vi "DG535.ProcCases.vi"(0 "i ref in":refnum<vi>, 1 "selector":string, 2 "Data":T1, 3 "call cluster":T2={"Object"="", "Selector"="", "CallType"=enum."synchronous", "Async Object"="", "Async Selector"="", "Data Descriptor"="", "Data"=[], "Error #"=0, "Expire"=0}, 5 "error in (no error)":errorcluster) -> (14 "i ref out":refnum<vi>, 17 "answer cluster":T2={"Object"="", "Selector"="", "CallType"=enum."synchronous", "Async Object"="", "Async Selector"="", "Data Descriptor"="", "Data"=[], "Error #"=0, "Expire"=0}, 19 "error out":errorcluster)   [LabVIEW 2014, in "DG535.lvlib"]
doc: "This method is called by a process from within the default case in the event loop. The methods of a class that are linked to events will be called from THIS method. Add your code here."
uses:
  DG535.lvlib
  CSCore/BaseProcess/BaseProcess.lvlib
  CSCore/CSSystem/CoreLib/CoreLib.lvlib
  CSCore/CSSystem/CoreLib/CoreLib.string 2 byte array.vi
  CSCore/CSSystem/CoreLib/CoreLib.double 2 byte array.vi
  CSCore/CSSystem/CoreLib/CoreLib.int 2 byte array.vi
  CSCore/CSSystem/CoreLib/CoreLib.byte array 2 int.vi
  CSCore/CSSystem/CoreLib/CoreLib.byte array 2 double.vi
  CSCore/CSSystem/CoreLib/CoreLib.byte array 2 short.vi
  CSCore/CSSystem/CoreLib/CoreLib.byte array 2 string.vi
  CSCore/CSSystem/CoreLib/CoreLib.short 2 byte array.vi
  CSCore/BaseProcess/BaseProcess.descriptor string definition.ctl
  CSCore/CSSystem/CoreDefs/CoreDefs.call_type.ctl
  CSCore/CSSystem/CoreDefs/CoreDefs.rawDataType.ctl
panel:
  in  "error IO":errorcluster
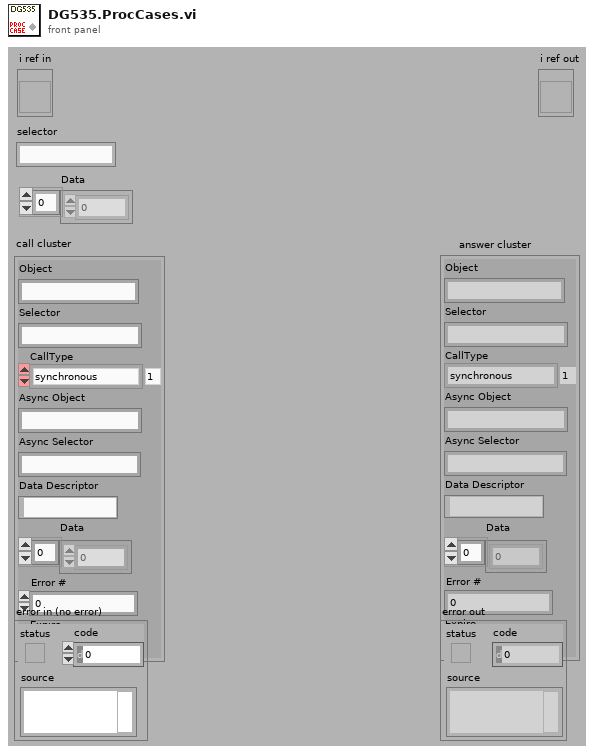
[diagram p1: front panel]
types:
  T1 = typedef "CoreDefs.rawDataType.ctl" = i8[]
  T2 = typedef "CoreDefs.call_type.ctl" = cluster{"Object":string, "Selector":string, "CallType":enum16{"simple", "synchronous", "asynchronous"}, "Async Object":string, "Async Selector":string, "Data Descriptor":T3, "Data":T1, "Error #":i32, "Expire":u32}
  T3 = typedef "BaseProcess.lvlib/BaseProcess.descriptor string definition.ctl" = string
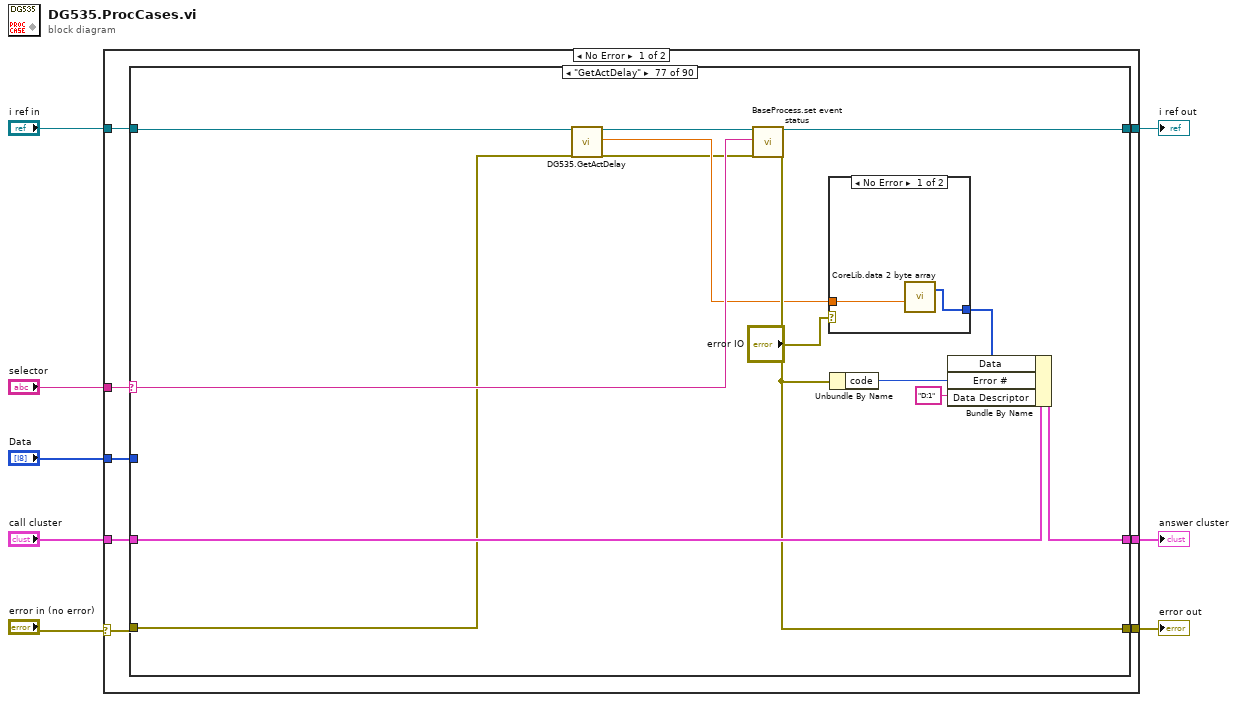
[diagram p0: block diagram]
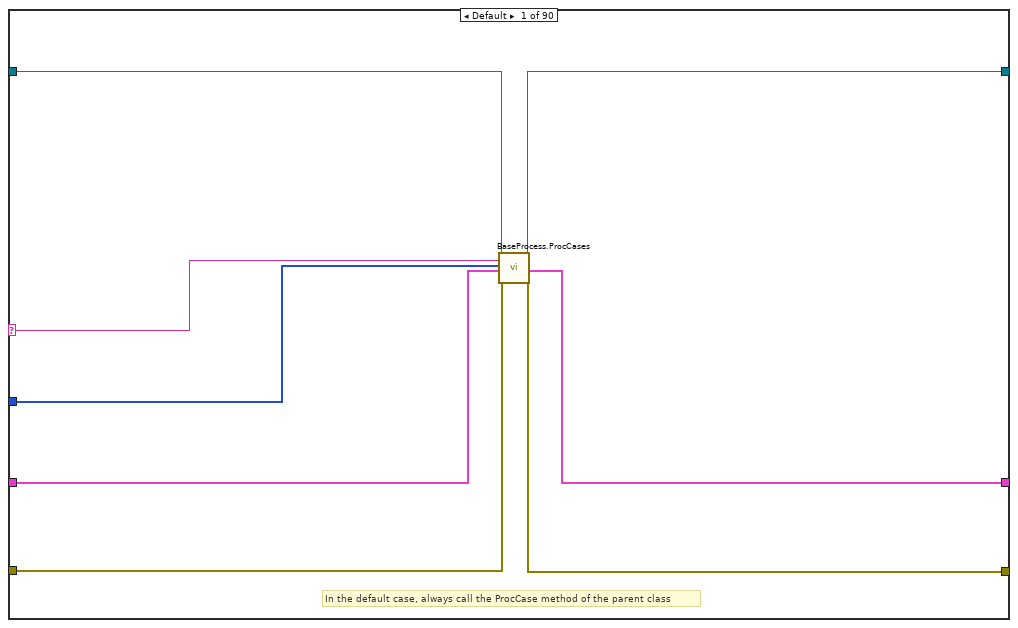
[diagram p2: hidden frame]
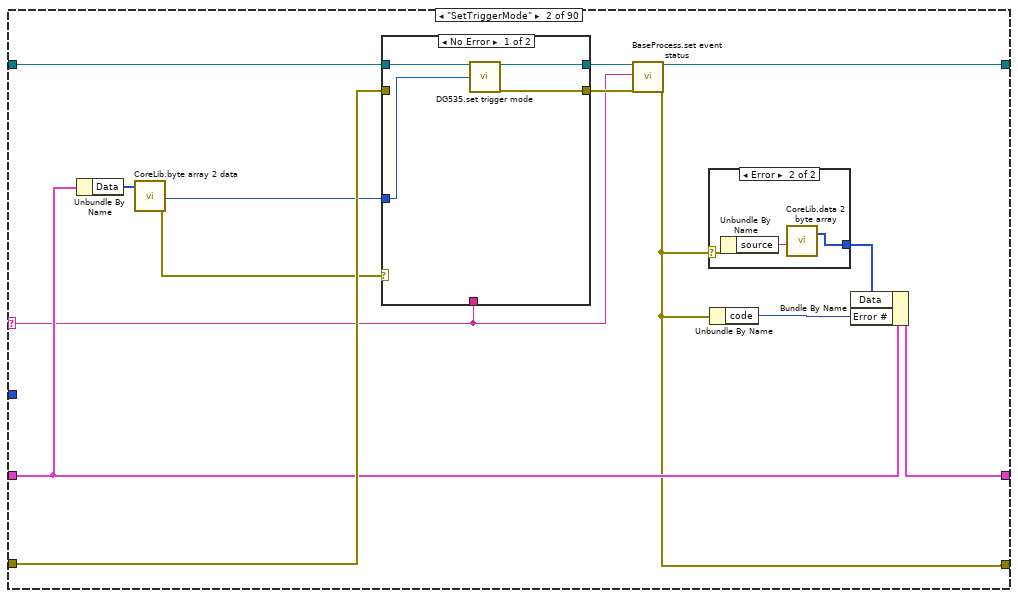
[diagram p3: hidden frame]
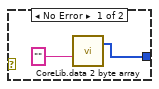
[diagram p4: hidden frame]
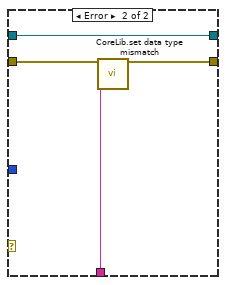
[diagram p5: hidden frame]
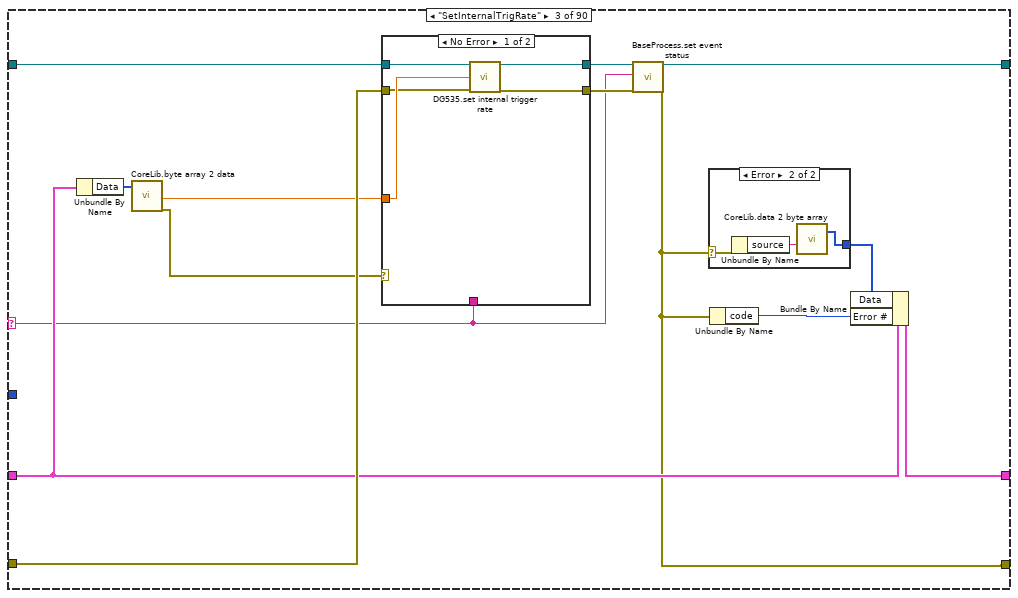
[diagram p6: hidden frame]
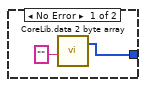
[diagram p7: hidden frame]
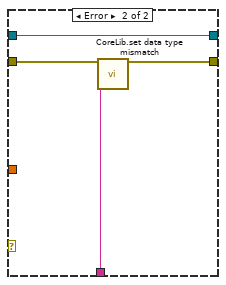
[diagram p8: hidden frame]
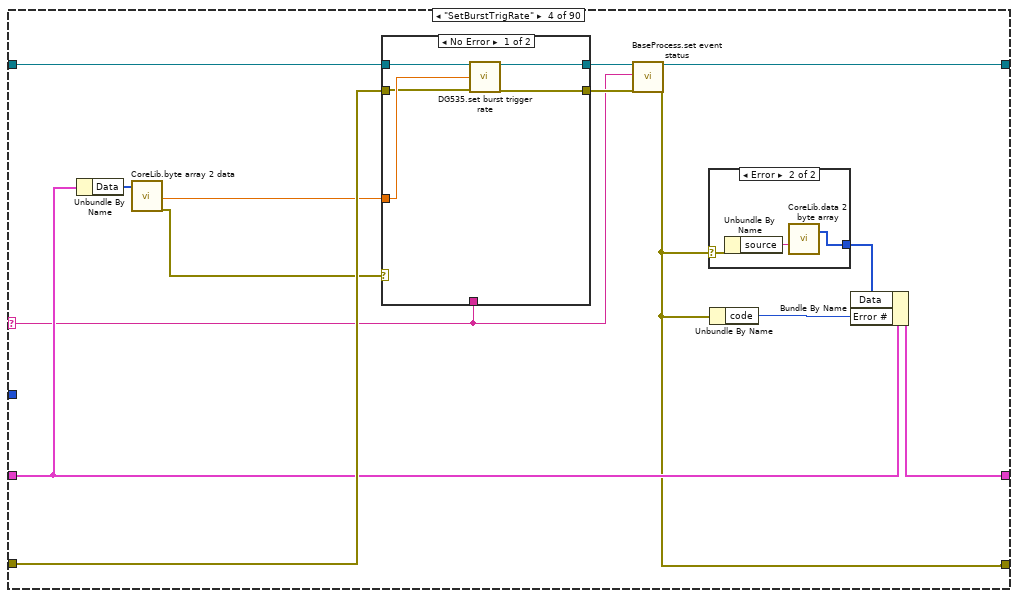
[diagram p9: hidden frame]
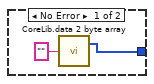
[diagram p10: hidden frame]
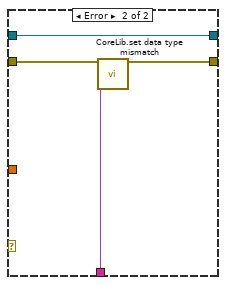
[diagram p11: hidden frame]
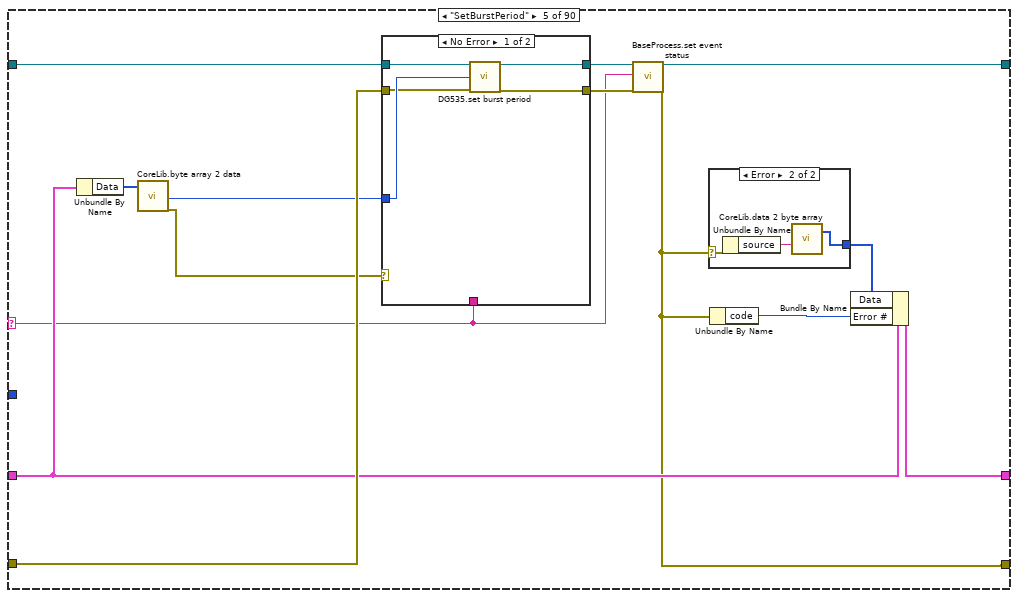
[diagram p12: hidden frame]
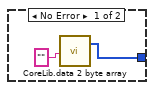
[diagram p13: hidden frame]
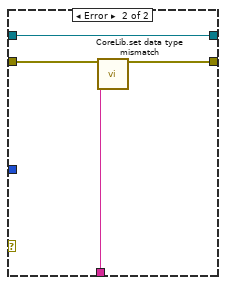
[diagram p14: hidden frame]
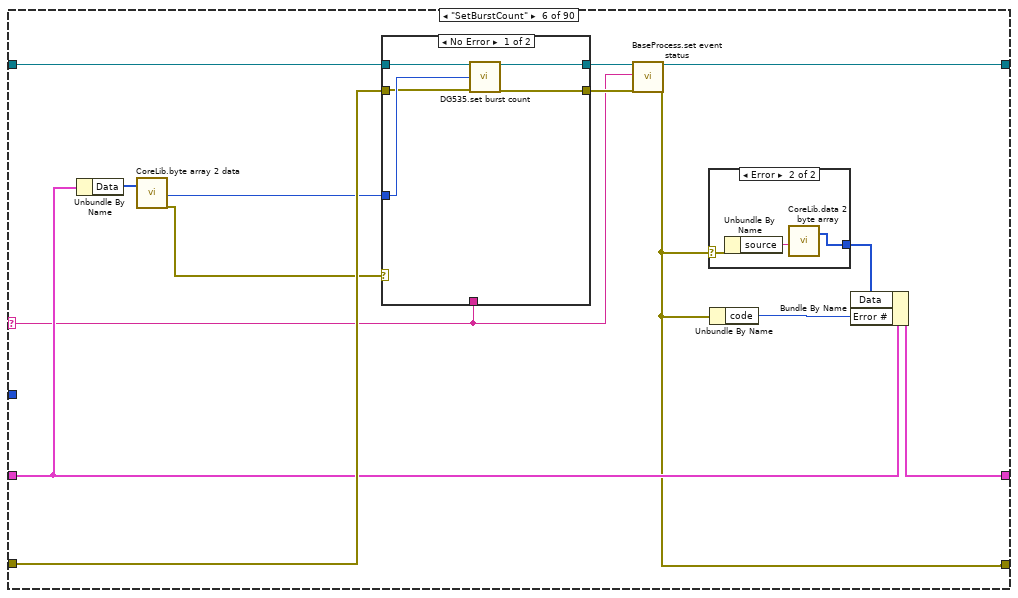
[diagram p15: hidden frame]
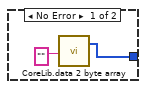
[diagram p16: hidden frame]
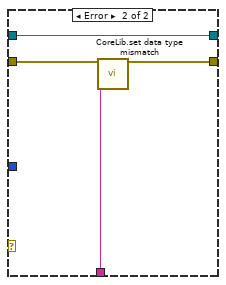
[diagram p17: hidden frame]
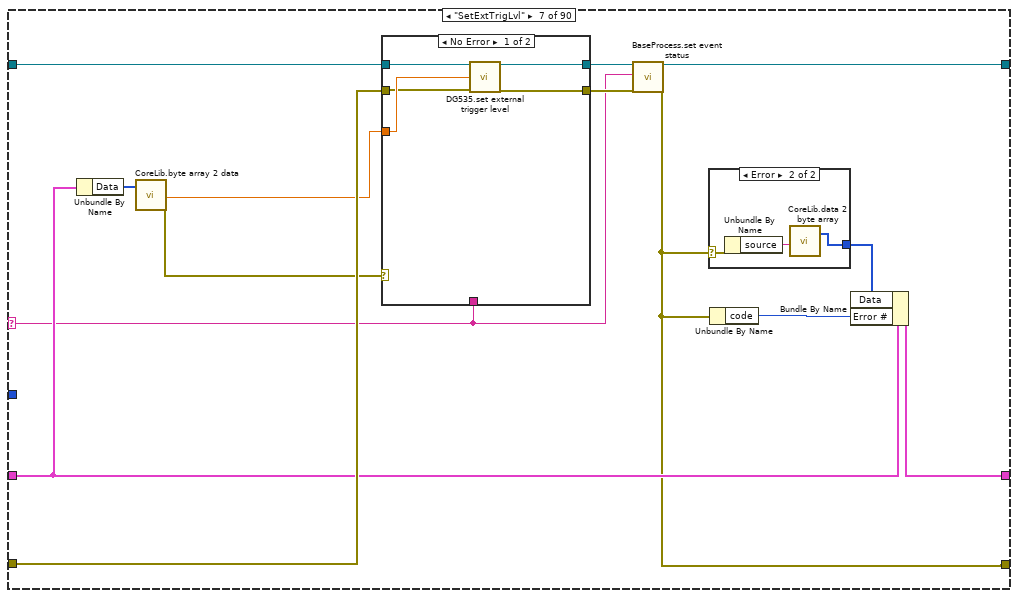
[diagram p18: hidden frame]
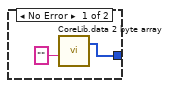
[diagram p19: hidden frame]
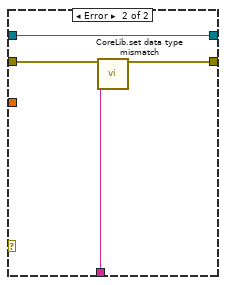
[diagram p20: hidden frame]
diagram:
  n1 = case shown="No Error" "error in (no error)" {
    selector: "error in (no error)" -> [w9 w2268]
    tunnel: "selector" -> [w16 _]
    tunnel: [w15 w2267] -> w7
    tunnel: "call cluster" -> [w14 w2267]
    tunnel: "i ref in" -> [w13 w2269]
    tunnel: [w12 w2269] -> w4
    tunnel: [w11 w2268] -> w3
    tunnel: "Data" -> [w10 _]
    frame No Error {
      n2 = case shown="\"GetActDelay\"" w16 {
        selector: w16 -> [w18 w30 w57 w85 w113 w141 w169 w201 w233 w261 w289 w317 w345 w373 w401 w429 w461 w493 w521 w549 w577 w605 w633 w661 w689 w717 w745 w773 w801 w829 w857 w885 w917 w949 w981 w1013 w1045 w1077 w1109 w1133 w1168 w1200 w1232 w1264 w1296 w1315 w1334 w1353 w1372 w1391 w1410 w1429 w1448 w1467 w1485 w1503 w1521 w1539 w1557 w1575 w1593 w1611 w1629 w1647 w1665 w1683 w1701 w1719 w1737 w1755 w1773 w1791 w1809 w1827 w1863 w1928 w1967 w1985 w2006 w2027 w2047 w2077 w2128 w2147 w2166 w2184 w2202 w2221 w2239 w2257]
        tunnel: w10 -> [w19 _ _ _ _ _ _ _ _ _ _ _ _ _ _ _ _ _ _ _ _ _ _ _ _ _ _ _ _ _ _ _ _ _ _ _ _ _ _ _ _ _ _ _ _ _ _ _ _ _ _ _ _ _ _ _ _ _ _ _ _ _ _ _ _ _ _ _ _ _ _ _ _ _ _ _ _ _ _ _ _ _ _ _ _ _ _ _ _ _]
        tunnel: w13 -> [w17 w38 w65 w93 w121 w149 w177 w209 w241 w269 w297 w325 w353 w381 w409 w437 w469 w501 w529 w557 w585 w613 w641 w669 w697 w725 w753 w781 w809 w837 w865 w893 w925 w957 w989 w1021 w1053 w1085 w1117 w1144 w1176 w1208 w1240 w1272 w1293 w1312 w1331 w1350 w1369 w1388 w1407 w1426 w1445 w1464 w1482 w1500 w1518 w1536 w1554 w1572 w1590 w1608 w1626 w1644 w1662 w1680 w1698 w1716 w1734 w1752 w1770 w1788 w1806 w1824 w1871 w1936 w1961 w1983 w2004 w2025 w2045 w2085 w2125 w2144 w2163 w2181 w2199 w2218 w2236 w2254]
        tunnel: [w24 w29 w56 w84 w112 w140 w168 w200 w232 w260 w288 w316 w344 w372 w400 w428 w460 w492 w520 w548 w576 w604 w632 w660 w688 w716 w744 w772 w800 w828 w856 w884 w916 w948 w980 w1012 w1044 w1076 w1108 w1138 w1167 w1199 w1231 w1263 w1295 w1314 w1333 w1352 w1371 w1390 w1409 w1428 w1447 w1466 w1484 w1502 w1520 w1538 w1556 w1574 w1592 w1610 w1628 w1646 w1664 w1682 w1700 w1718 w1736 w1754 w1772 w1790 w1808 w1826 w1862 w1927 w1963 w1984 w2005 w2026 w2046 w2076 w2127 w2146 w2165 w2183 w2201 w2220 w2238 w2256] -> w12
        tunnel: w14 -> [w20 w35 w62 w90 w118 w146 w174 w206 w238 w266 w294 w322 w350 w378 w406 w434 w466 w498 w526 w554 w582 w610 w638 w666 w694 w722 w750 w778 w806 w834 w862 w890 w922 w954 w986 w1018 w1050 w1082 w1114 w1141 w1173 w1205 w1237 w1269 w1299 w1318 w1337 w1356 w1375 w1394 w1413 w1432 w1451 w1470 w1488 w1506 w1524 w1542 w1560 w1578 w1596 w1614 w1632 w1650 w1668 w1686 w1704 w1722 w1740 w1758 w1776 w1794 w1812 w1830 w1868 w1933 w1966 w1988 w2009 w2030 w2050 w2082 w2132 w2151 w2170 w2188 w2206 w2224 w2242 w2260]
        tunnel: [w21 w34 w61 w89 w117 w145 w173 w205 w237 w265 w293 w321 w349 w377 w405 w433 w465 w497 w525 w553 w581 w609 w637 w665 w693 w721 w749 w777 w805 w833 w861 w889 w921 w953 w985 w1017 w1049 w1081 w1113 w1135 w1172 w1204 w1236 w1268 w1298 w1317 w1336 w1355 w1374 w1393 w1412 w1431 w1450 w1469 w1487 w1505 w1523 w1541 w1559 w1577 w1595 w1613 w1631 w1649 w1667 w1685 w1703 w1721 w1739 w1757 w1775 w1793 w1811 w1829 w1867 w1932 w1965 w1987 w2008 w2029 w2049 w2081 w2131 w2150 w2169 w2187 w2205 w2223 w2241 w2259] -> w15
        tunnel: w9 -> [w23 w37 w64 w92 w120 w148 w176 w208 w240 w268 w296 w324 w352 w380 w408 w436 w468 w500 w528 w556 w584 w612 w640 w668 w696 w724 w752 w780 w808 w836 w864 w892 w924 w956 w988 w1020 w1052 w1084 w1116 w1143 w1175 w1207 w1239 w1271 w1294 w1313 w1332 w1351 w1370 w1389 w1408 w1427 w1446 w1465 w1483 w1501 w1519 w1537 w1555 w1573 w1591 w1609 w1627 w1645 w1663 w1681 w1699 w1717 w1735 w1753 w1771 w1789 w1807 w1825 w1870 w1935 w1962 w1982 w2003 w2024 w2044 w2084 w2126 w2145 w2164 w2182 w2200 w2219 w2237 w2255]
        tunnel: [w22 w31 w58 w86 w114 w142 w170 w202 w234 w262 w290 w318 w346 w374 w402 w430 w462 w494 w522 w550 w578 w606 w634 w662 w690 w718 w746 w774 w802 w830 w858 w886 w918 w950 w982 w1014 w1046 w1078 w1110 w1136 w1169 w1201 w1233 w1265 w1297 w1316 w1335 w1354 w1373 w1392 w1411 w1430 w1449 w1468 w1486 w1504 w1522 w1540 w1558 w1576 w1594 w1612 w1630 w1648 w1666 w1684 w1702 w1720 w1738 w1756 w1774 w1792 w1810 w1828 w1864 w1929 w1964 w1986 w2007 w2028 w2048 w2078 w2129 w2148 w2167 w2185 w2203 w2222 w2240 w2258] -> w11
        frame Default {
          # "In the default case, always call the ProcCase method of the parent class"
          n3 = call "BaseProcess.ProcCases.vi"("i ref in"=w17, "selector"=w18, "Data"=w19, "call cluster"=w20, "error in (no error)"=w23) -> ("i ref out"=w24:refnum<vi>, "answer cluster"=w21:T2, "error out"=w22:errorcluster)  [unwired: 12 in]
        }
        frame "SetTriggerMode" {
          n4 = Unbundle By Name(w35) -> ("Data"=w28:T1)
          n5 = call-poly "CoreLib.byte array 2 data.vi"("byteArray"=w28) -> ("i32"=w27:i32, "error out"=w26:errorcluster)  [unwired: 16 in, 1 out]
          n6 = case shown="No Error" w26 {
            tunnel: [w45 w51] -> w33
            tunnel: w38 -> [w46 w51]
            tunnel: w37 -> [_ w50]
            tunnel: [w44 w49] -> w32
            tunnel: w30 -> [_ w48]
            tunnel: w27 -> [w47 _]
            frame No Error {
              n7 = call "DG535.set trigger mode.vi"("i ref in"=w46, "Trigger Mode"=w47) -> ("i ref out"=w45:refnum<vi>, "error out"=w44:errorcluster)  [unwired: 12 in]
            }
            frame Error {
              n8 = call "CoreLib.set data type mismatch.vi"("error in (no error)"=w50, "error source"=w48) -> ("error out"=w49:errorcluster)  [unwired: 17 in]
            }
          }
          n9 = call "BaseProcess.set event status.vi"("i ref in"=w33, "EventStatus"=w30, "error in (no error)"=w32) -> ("i ref out"=w29:refnum<vi>, "error out"=w31:errorcluster)  [unwired: 14 in, 1 out]
          n10 = case shown="Error" w31 {
            selector: w31 -> [_ w43]
            tunnel: [w39 w41] -> w25
            frame No Error {
              n11 = call-poly "CoreLib.data 2 byte array.vi"("string"="" ("source")) -> ("byteArray out"=w39:T1)  [unwired: 18 in]
            }
            frame Error {
              n12 = Unbundle By Name(w43) -> ("source"=w42:string)
              n13 = call-poly "CoreLib.data 2 byte array.vi"("string"=w42) -> ("byteArray out"=w41:T1)  [unwired: 18 in]
            }
          }
          n14 = Unbundle By Name(w31) -> ("code"=w36:i32)
          n15 = Bundle By Name(cluster=w35, "Data"=w25, "Error #"=w36) -> (w34:T2)
        }
        frame "SetInternalTrigRate" {
          n16 = Unbundle By Name(w62) -> ("Data"=w55:T1)
          n17 = call-poly "CoreLib.byte array 2 data.vi"("byteArray"=w55) -> ("d64"=w54:dbl, "error out"=w53:errorcluster)  [unwired: 16 in, 1 out]
          n18 = case shown="No Error" w53 {
            tunnel: [w73 w79] -> w60
            tunnel: w65 -> [w74 w79]
            tunnel: w64 -> [w71 w78]
            tunnel: [w72 w77] -> w59
            tunnel: w57 -> [_ w76]
            tunnel: w54 -> [w75 _]
            frame No Error {
              n19 = call "DG535.set internal trigger rate.vi"("i ref in"=w74, "internal trigger rate"=w75, "error in (no error)"=w71) -> ("i ref out"=w73:refnum<vi>, "error out"=w72:errorcluster)  [unwired: 11 in]
            }
            frame Error {
              n20 = call "CoreLib.set data type mismatch.vi"("error in (no error)"=w78, "error source"=w76) -> ("error out"=w77:errorcluster)  [unwired: 17 in]
            }
          }
          n21 = call "BaseProcess.set event status.vi"("i ref in"=w60, "EventStatus"=w57, "error in (no error)"=w59) -> ("i ref out"=w56:refnum<vi>, "error out"=w58:errorcluster)  [unwired: 14 in, 1 out]
          n22 = case shown="Error" w58 {
            selector: w58 -> [_ w70]
            tunnel: [w66 w68] -> w52
            frame No Error {
              n23 = call-poly "CoreLib.data 2 byte array.vi"("string"="" ("source")) -> ("byteArray out"=w66:T1)  [unwired: 18 in]
            }
            frame Error {
              n24 = Unbundle By Name(w70) -> ("source"=w69:string)
              n25 = call-poly "CoreLib.data 2 byte array.vi"("string"=w69) -> ("byteArray out"=w68:T1)  [unwired: 18 in]
            }
          }
          n26 = Unbundle By Name(w58) -> ("code"=w63:i32)
          n27 = Bundle By Name(cluster=w62, "Data"=w52, "Error #"=w63) -> (w61:T2)
        }
        frame "SetBurstTrigRate" {
          n28 = Unbundle By Name(w90) -> ("Data"=w83:T1)
          n29 = call-poly "CoreLib.byte array 2 data.vi"("byteArray"=w83) -> ("d64"=w82:dbl, "error out"=w81:errorcluster)  [unwired: 16 in, 1 out]
          n30 = case shown="No Error" w81 {
            tunnel: [w99 w107] -> w88
            tunnel: w93 -> [w102 w107]
            tunnel: w92 -> [w100 w106]
            tunnel: [w101 w105] -> w87
            tunnel: w85 -> [_ w104]
            tunnel: w82 -> [w103 _]
            frame No Error {
              n31 = call "DG535.set burst trigger rate.vi"("i ref in"=w102, "Burst trigger rate"=w103, "error in (no error)"=w100) -> ("i ref out"=w99:refnum<vi>, "error out"=w101:errorcluster)  [unwired: 11 in]
            }
            frame Error {
              n32 = call "CoreLib.set data type mismatch.vi"("error in (no error)"=w106, "error source"=w104) -> ("error out"=w105:errorcluster)  [unwired: 17 in]
            }
          }
          n33 = call "BaseProcess.set event status.vi"("i ref in"=w88, "EventStatus"=w85, "error in (no error)"=w87) -> ("i ref out"=w84:refnum<vi>, "error out"=w86:errorcluster)  [unwired: 14 in, 1 out]
          n34 = case shown="Error" w86 {
            selector: w86 -> [_ w98]
            tunnel: [w94 w96] -> w80
            frame No Error {
              n35 = call-poly "CoreLib.data 2 byte array.vi"("string"="" ("source")) -> ("byteArray out"=w94:T1)  [unwired: 18 in]
            }
            frame Error {
              n36 = Unbundle By Name(w98) -> ("source"=w97:string)
              n37 = call-poly "CoreLib.data 2 byte array.vi"("string"=w97) -> ("byteArray out"=w96:T1)  [unwired: 18 in]
            }
          }
          n38 = Unbundle By Name(w86) -> ("code"=w91:i32)
          n39 = Bundle By Name(cluster=w90, "Data"=w80, "Error #"=w91) -> (w89:T2)
        }
        frame "SetBurstPeriod" {
          n40 = Unbundle By Name(w118) -> ("Data"=w111:T1)
          n41 = call-poly "CoreLib.byte array 2 data.vi"("byteArray"=w111) -> ("i32"=w110:i32, "error out"=w109:errorcluster)  [unwired: 16 in, 1 out]
          n42 = case shown="No Error" w109 {
            tunnel: [w127 w135] -> w116
            tunnel: w121 -> [w130 w135]
            tunnel: w120 -> [w128 w134]
            tunnel: [w129 w133] -> w115
            tunnel: w113 -> [_ w132]
            tunnel: w110 -> [w131 _]
            frame No Error {
              n43 = call "DG535.set burst period.vi"("i ref in"=w130, "burst period"=w131, "error in (no error)"=w128) -> ("i ref out"=w127:refnum<vi>, "error out"=w129:errorcluster)  [unwired: 11 in]
            }
            frame Error {
              n44 = call "CoreLib.set data type mismatch.vi"("error in (no error)"=w134, "error source"=w132) -> ("error out"=w133:errorcluster)  [unwired: 17 in]
            }
          }
          n45 = call "BaseProcess.set event status.vi"("i ref in"=w116, "EventStatus"=w113, "error in (no error)"=w115) -> ("i ref out"=w112:refnum<vi>, "error out"=w114:errorcluster)  [unwired: 14 in, 1 out]
          n46 = case shown="Error" w114 {
            selector: w114 -> [_ w126]
            tunnel: [w122 w124] -> w108
            frame No Error {
              n47 = call-poly "CoreLib.data 2 byte array.vi"("string"="" ("source")) -> ("byteArray out"=w122:T1)  [unwired: 18 in]
            }
            frame Error {
              n48 = Unbundle By Name(w126) -> ("source"=w125:string)
              n49 = call-poly "CoreLib.data 2 byte array.vi"("string"=w125) -> ("byteArray out"=w124:T1)  [unwired: 18 in]
            }
          }
          n50 = Unbundle By Name(w114) -> ("code"=w119:i32)
          n51 = Bundle By Name(cluster=w118, "Data"=w108, "Error #"=w119) -> (w117:T2)
        }
        frame "SetBurstCount" {
          n52 = Unbundle By Name(w146) -> ("Data"=w139:T1)
          n53 = call-poly "CoreLib.byte array 2 data.vi"("byteArray"=w139) -> ("i32"=w138:i32, "error out"=w137:errorcluster)  [unwired: 16 in, 1 out]
          n54 = case shown="No Error" w137 {
            tunnel: [w155 w163] -> w144
            tunnel: w149 -> [w158 w163]
            tunnel: w148 -> [w156 w162]
            tunnel: [w157 w161] -> w143
            tunnel: w141 -> [_ w160]
            tunnel: w138 -> [w159 _]
            frame No Error {
              n55 = call "DG535.set burst count.vi"("i ref in"=w158, "burst count"=w159, "error in (no error)"=w156) -> ("i ref out"=w155:refnum<vi>, "error out"=w157:errorcluster)  [unwired: 11 in]
            }
            frame Error {
              n56 = call "CoreLib.set data type mismatch.vi"("error in (no error)"=w162, "error source"=w160) -> ("error out"=w161:errorcluster)  [unwired: 17 in]
            }
          }
          n57 = call "BaseProcess.set event status.vi"("i ref in"=w144, "EventStatus"=w141, "error in (no error)"=w143) -> ("i ref out"=w140:refnum<vi>, "error out"=w142:errorcluster)  [unwired: 14 in, 1 out]
          n58 = case shown="Error" w142 {
            selector: w142 -> [_ w154]
            tunnel: [w150 w152] -> w136
            frame No Error {
              n59 = call-poly "CoreLib.data 2 byte array.vi"("string"="" ("source")) -> ("byteArray out"=w150:T1)  [unwired: 18 in]
            }
            frame Error {
              n60 = Unbundle By Name(w154) -> ("source"=w153:string)
              n61 = call-poly "CoreLib.data 2 byte array.vi"("string"=w153) -> ("byteArray out"=w152:T1)  [unwired: 18 in]
            }
          }
          n62 = Unbundle By Name(w142) -> ("code"=w147:i32)
          n63 = Bundle By Name(cluster=w146, "Data"=w136, "Error #"=w147) -> (w145:T2)
        }
        frame "SetExtTrigLvl" {
          n64 = Unbundle By Name(w174) -> ("Data"=w167:T1)
          n65 = call-poly "CoreLib.byte array 2 data.vi"("byteArray"=w167) -> ("d64"=w166:dbl, "error out"=w165:errorcluster)  [unwired: 16 in, 1 out]
          n66 = case shown="No Error" w165 {
            tunnel: [w183 w191] -> w172
            tunnel: w177 -> [w186 w191]
            tunnel: w176 -> [w184 w190]
            tunnel: [w185 w189] -> w171
            tunnel: w169 -> [_ w188]
            tunnel: w166 -> [w187 _]
            frame No Error {
              n67 = call "DG535.set external trigger level.vi"("i ref in"=w186, "external trigger level"=w187, "error in (no error)"=w184) -> ("i ref out"=w183:refnum<vi>, "error out"=w185:errorcluster)  [unwired: 11 in]
            }
            frame Error {
              n68 = call "CoreLib.set data type mismatch.vi"("error in (no error)"=w190, "error source"=w188) -> ("error out"=w189:errorcluster)  [unwired: 17 in]
            }
          }
          n69 = call "BaseProcess.set event status.vi"("i ref in"=w172, "EventStatus"=w169, "error in (no error)"=w171) -> ("i ref out"=w168:refnum<vi>, "error out"=w170:errorcluster)  [unwired: 14 in, 1 out]
          n70 = case shown="Error" w170 {
            selector: w170 -> [_ w182]
            tunnel: [w178 w180] -> w164
            frame No Error {
              n71 = call-poly "CoreLib.data 2 byte array.vi"("string"="" ("source")) -> ("byteArray out"=w178:T1)  [unwired: 18 in]
            }
            frame Error {
              n72 = Unbundle By Name(w182) -> ("source"=w181:string)
              n73 = call-poly "CoreLib.data 2 byte array.vi"("string"=w181) -> ("byteArray out"=w180:T1)  [unwired: 18 in]
            }
          }
          n74 = Unbundle By Name(w170) -> ("code"=w175:i32)
          n75 = Bundle By Name(cluster=w174, "Data"=w164, "Error #"=w175) -> (w173:T2)
        }
        frame "SetTriggerSlope" {
          n76 = Unbundle By Name(w206) -> ("Data"=w199:T1)
          n77 = call-poly "CoreLib.byte array 2 data.vi"("byteArray"=w199) -> ("i16"=w194:i16, "error out"=w193:errorcluster)  [unwired: 16 in, 1 out]
          n78 = Equal To 0?(x=w194) -> (x = 0?=w196:bool)
          n79 = Select(t=FALSE, s=w196, f=TRUE) -> (s? t:f=w195:bool)
          n80 = case shown="No Error" w193 {
            tunnel: [w215 w223] -> w204
            tunnel: w209 -> [w218 w223]
            tunnel: w208 -> [w216 w222]
            tunnel: [w217 w221] -> w203
            tunnel: w201 -> [_ w220]
            tunnel: w195 -> [w219 _]
            frame No Error {
              n81 = call "DG535.set trigger slope.vi"("i ref in"=w218, "trigger slope"=w219, "error in (no error)"=w216) -> ("i ref out"=w215:refnum<vi>, "error out"=w217:errorcluster)  [unwired: 11 in]
            }
            frame Error {
              n82 = call "CoreLib.set data type mismatch.vi"("error in (no error)"=w222, "error source"=w220) -> ("error out"=w221:errorcluster)  [unwired: 17 in]
            }
          }
          n83 = call "BaseProcess.set event status.vi"("i ref in"=w204, "EventStatus"=w201, "error in (no error)"=w203) -> ("i ref out"=w200:refnum<vi>, "error out"=w202:errorcluster)  [unwired: 14 in, 1 out]
          n84 = case shown="Error" w202 {
            selector: w202 -> [_ w214]
            tunnel: [w210 w212] -> w192
            frame No Error {
              n85 = call-poly "CoreLib.data 2 byte array.vi"("string"="" ("source")) -> ("byteArray out"=w210:T1)  [unwired: 18 in]
            }
            frame Error {
              n86 = Unbundle By Name(w214) -> ("source"=w213:string)
              n87 = call-poly "CoreLib.data 2 byte array.vi"("string"=w213) -> ("byteArray out"=w212:T1)  [unwired: 18 in]
            }
          }
          n88 = Unbundle By Name(w202) -> ("code"=w207:i32)
          n89 = Bundle By Name(cluster=w206, "Data"=w192, "Error #"=w207) -> (w205:T2)
        }
        frame "SetInputImpedance" {
          n90 = Unbundle By Name(w238) -> ("Data"=w227:T1)
          n91 = call-poly "CoreLib.byte array 2 data.vi"("byteArray"=w227) -> ("i16"=w226:i16, "error out"=w225:errorcluster)  [unwired: 16 in, 1 out]
          n92 = Equal To 0?(x=w226) -> (x = 0?=w229:bool)
          n93 = Select(t=FALSE, s=w229, f=TRUE) -> (s? t:f=w228:bool)
          n94 = case shown="No Error" w225 {
            tunnel: [w247 w255] -> w236
            tunnel: w241 -> [w250 w255]
            tunnel: w240 -> [w248 w254]
            tunnel: [w249 w253] -> w235
            tunnel: w233 -> [_ w252]
            tunnel: w228 -> [w251 _]
            frame No Error {
              n95 = call "DG535.set input impedance.vi"("i ref in"=w250, "input impedance"=w251, "error in (no error)"=w248) -> ("i ref out"=w247:refnum<vi>, "error out"=w249:errorcluster)  [unwired: 11 in]
            }
            frame Error {
              n96 = call "CoreLib.set data type mismatch.vi"("error in (no error)"=w254, "error source"=w252) -> ("error out"=w253:errorcluster)  [unwired: 17 in]
            }
          }
          n97 = call "BaseProcess.set event status.vi"("i ref in"=w236, "EventStatus"=w233, "error in (no error)"=w235) -> ("i ref out"=w232:refnum<vi>, "error out"=w234:errorcluster)  [unwired: 14 in, 1 out]
          n98 = case shown="Error" w234 {
            selector: w234 -> [_ w246]
            tunnel: [w242 w244] -> w224
            frame No Error {
              n99 = call-poly "CoreLib.data 2 byte array.vi"("string"="" ("source")) -> ("byteArray out"=w242:T1)  [unwired: 18 in]
            }
            frame Error {
              n100 = Unbundle By Name(w246) -> ("source"=w245:string)
              n101 = call-poly "CoreLib.data 2 byte array.vi"("string"=w245) -> ("byteArray out"=w244:T1)  [unwired: 18 in]
            }
          }
          n102 = Unbundle By Name(w234) -> ("code"=w239:i32)
          n103 = Bundle By Name(cluster=w238, "Data"=w224, "Error #"=w239) -> (w237:T2)
        }
        frame "SetT0Mode" {
          n104 = Unbundle By Name(w266) -> ("Data"=w259:T1)
          n105 = call-poly "CoreLib.byte array 2 data.vi"("byteArray"=w259) -> ("i32"=w258:i32, "error out"=w257:errorcluster)  [unwired: 16 in, 1 out]
          n106 = case shown="No Error" w257 {
            tunnel: [w275 w283] -> w264
            tunnel: w269 -> [w278 w283]
            tunnel: w268 -> [w276 w282]
            tunnel: [w277 w281] -> w263
            tunnel: w261 -> [_ w280]
            tunnel: w258 -> [w279 _]
            frame No Error {
              n107 = call "DG535.set T0 mode.vi"("i ref in"=w278, "mode"=w279, "error in"=w276) -> ("i ref out"=w275:refnum<vi>, "error out"=w277:errorcluster)  [unwired: 11 in]
            }
            frame Error {
              n108 = call "CoreLib.set data type mismatch.vi"("error in (no error)"=w282, "error source"=w280) -> ("error out"=w281:errorcluster)  [unwired: 17 in]
            }
          }
          n109 = call "BaseProcess.set event status.vi"("i ref in"=w264, "EventStatus"=w261, "error in (no error)"=w263) -> ("i ref out"=w260:refnum<vi>, "error out"=w262:errorcluster)  [unwired: 14 in, 1 out]
          n110 = case shown="Error" w262 {
            selector: w262 -> [_ w274]
            tunnel: [w270 w272] -> w256
            frame No Error {
              n111 = call-poly "CoreLib.data 2 byte array.vi"("string"="" ("source")) -> ("byteArray out"=w270:T1)  [unwired: 18 in]
            }
            frame Error {
              n112 = Unbundle By Name(w274) -> ("source"=w273:string)
              n113 = call-poly "CoreLib.data 2 byte array.vi"("string"=w273) -> ("byteArray out"=w272:T1)  [unwired: 18 in]
            }
          }
          n114 = Unbundle By Name(w262) -> ("code"=w267:i32)
          n115 = Bundle By Name(cluster=w266, "Data"=w256, "Error #"=w267) -> (w265:T2)
        }
        frame "SetAMode" {
          n116 = Unbundle By Name(w294) -> ("Data"=w287:T1)
          n117 = call-poly "CoreLib.byte array 2 data.vi"("byteArray"=w287) -> ("i32"=w286:i32, "error out"=w285:errorcluster)  [unwired: 16 in, 1 out]
          n118 = case shown="No Error" w285 {
            tunnel: [w303 w311] -> w292
            tunnel: w297 -> [w306 w311]
            tunnel: w296 -> [w304 w310]
            tunnel: [w305 w309] -> w291
            tunnel: w289 -> [_ w308]
            tunnel: w286 -> [w307 _]
            frame No Error {
              n119 = call "DG535.set A mode.vi"("i ref in"=w306, "mode"=w307, "error in"=w304) -> ("i ref out"=w303:refnum<vi>, "error out"=w305:errorcluster)  [unwired: 11 in]
            }
            frame Error {
              n120 = call "CoreLib.set data type mismatch.vi"("error in (no error)"=w310, "error source"=w308) -> ("error out"=w309:errorcluster)  [unwired: 17 in]
            }
          }
          n121 = call "BaseProcess.set event status.vi"("i ref in"=w292, "EventStatus"=w289, "error in (no error)"=w291) -> ("i ref out"=w288:refnum<vi>, "error out"=w290:errorcluster)  [unwired: 14 in, 1 out]
          n122 = case shown="Error" w290 {
            selector: w290 -> [_ w302]
            tunnel: [w298 w300] -> w284
            frame No Error {
              n123 = call-poly "CoreLib.data 2 byte array.vi"("string"="" ("source")) -> ("byteArray out"=w298:T1)  [unwired: 18 in]
            }
            frame Error {
              n124 = Unbundle By Name(w302) -> ("source"=w301:string)
              n125 = call-poly "CoreLib.data 2 byte array.vi"("string"=w301) -> ("byteArray out"=w300:T1)  [unwired: 18 in]
            }
          }
          n126 = Unbundle By Name(w290) -> ("code"=w295:i32)
          n127 = Bundle By Name(cluster=w294, "Data"=w284, "Error #"=w295) -> (w293:T2)
        }
        frame "SetBMode" {
          n128 = Unbundle By Name(w322) -> ("Data"=w315:T1)
          n129 = call-poly "CoreLib.byte array 2 data.vi"("byteArray"=w315) -> ("i32"=w313:i32, "error out"=w314:errorcluster)  [unwired: 16 in, 1 out]
          n130 = case shown="No Error" w314 {
            tunnel: [w331 w339] -> w320
            tunnel: w325 -> [w334 w339]
            tunnel: w324 -> [w332 w338]
            tunnel: [w333 w337] -> w319
            tunnel: w317 -> [_ w336]
            tunnel: w313 -> [w335 _]
            frame No Error {
              n131 = call "DG535.set B mode.vi"("i ref in"=w334, "mode"=w335, "error in"=w332) -> ("i ref out"=w331:refnum<vi>, "error out"=w333:errorcluster)  [unwired: 11 in]
            }
            frame Error {
              n132 = call "CoreLib.set data type mismatch.vi"("error in (no error)"=w338, "error source"=w336) -> ("error out"=w337:errorcluster)  [unwired: 17 in]
            }
          }
          n133 = call "BaseProcess.set event status.vi"("i ref in"=w320, "EventStatus"=w317, "error in (no error)"=w319) -> ("i ref out"=w316:refnum<vi>, "error out"=w318:errorcluster)  [unwired: 14 in, 1 out]
          n134 = case shown="Error" w318 {
            selector: w318 -> [_ w330]
            tunnel: [w326 w328] -> w312
            frame No Error {
              n135 = call-poly "CoreLib.data 2 byte array.vi"("string"="" ("source")) -> ("byteArray out"=w326:T1)  [unwired: 18 in]
            }
            frame Error {
              n136 = Unbundle By Name(w330) -> ("source"=w329:string)
              n137 = call-poly "CoreLib.data 2 byte array.vi"("string"=w329) -> ("byteArray out"=w328:T1)  [unwired: 18 in]
            }
          }
          n138 = Unbundle By Name(w318) -> ("code"=w323:i32)
          n139 = Bundle By Name(cluster=w322, "Data"=w312, "Error #"=w323) -> (w321:T2)
        }
        frame "SetABMode" {
          n140 = Unbundle By Name(w350) -> ("Data"=w343:T1)
          n141 = call-poly "CoreLib.byte array 2 data.vi"("byteArray"=w343) -> ("i32"=w342:i32, "error out"=w341:errorcluster)  [unwired: 16 in, 1 out]
          n142 = case shown="No Error" w341 {
            tunnel: [w359 w367] -> w348
            tunnel: w353 -> [w362 w367]
            tunnel: w352 -> [w360 w366]
            tunnel: [w361 w365] -> w347
            tunnel: w345 -> [_ w364]
            tunnel: w342 -> [w363 _]
            frame No Error {
              n143 = call "DG535.set AB mode.vi"("i ref in"=w362, "mode"=w363, "error in"=w360) -> ("i ref out"=w359:refnum<vi>, "error out"=w361:errorcluster)  [unwired: 11 in]
            }
            frame Error {
              n144 = call "CoreLib.set data type mismatch.vi"("error in (no error)"=w366, "error source"=w364) -> ("error out"=w365:errorcluster)  [unwired: 17 in]
            }
          }
          n145 = call "BaseProcess.set event status.vi"("i ref in"=w348, "EventStatus"=w345, "error in (no error)"=w347) -> ("i ref out"=w344:refnum<vi>, "error out"=w346:errorcluster)  [unwired: 14 in, 1 out]
          n146 = case shown="Error" w346 {
            selector: w346 -> [_ w358]
            tunnel: [w354 w356] -> w340
            frame No Error {
              n147 = call-poly "CoreLib.data 2 byte array.vi"("string"="" ("source")) -> ("byteArray out"=w354:T1)  [unwired: 18 in]
            }
            frame Error {
              n148 = Unbundle By Name(w358) -> ("source"=w357:string)
              n149 = call-poly "CoreLib.data 2 byte array.vi"("string"=w357) -> ("byteArray out"=w356:T1)  [unwired: 18 in]
            }
          }
          n150 = Unbundle By Name(w346) -> ("code"=w351:i32)
          n151 = Bundle By Name(cluster=w350, "Data"=w340, "Error #"=w351) -> (w349:T2)
        }
        frame "SetCMode" {
          n152 = Unbundle By Name(w378) -> ("Data"=w371:T1)
          n153 = call-poly "CoreLib.byte array 2 data.vi"("byteArray"=w371) -> ("i32"=w370:i32, "error out"=w369:errorcluster)  [unwired: 16 in, 1 out]
          n154 = case shown="No Error" w369 {
            tunnel: [w387 w395] -> w376
            tunnel: w381 -> [w390 w395]
            tunnel: w380 -> [w388 w394]
            tunnel: [w389 w393] -> w375
            tunnel: w373 -> [_ w392]
            tunnel: w370 -> [w391 _]
            frame No Error {
              n155 = call "DG535.set C mode.vi"("i ref in"=w390, "mode"=w391, "error in"=w388) -> ("i ref out"=w387:refnum<vi>, "error out"=w389:errorcluster)  [unwired: 11 in]
            }
            frame Error {
              n156 = call "CoreLib.set data type mismatch.vi"("error in (no error)"=w394, "error source"=w392) -> ("error out"=w393:errorcluster)  [unwired: 17 in]
            }
          }
          n157 = call "BaseProcess.set event status.vi"("i ref in"=w376, "EventStatus"=w373, "error in (no error)"=w375) -> ("i ref out"=w372:refnum<vi>, "error out"=w374:errorcluster)  [unwired: 14 in, 1 out]
          n158 = case shown="Error" w374 {
            selector: w374 -> [_ w386]
            tunnel: [w382 w384] -> w368
            frame No Error {
              n159 = call-poly "CoreLib.data 2 byte array.vi"("string"="" ("source")) -> ("byteArray out"=w382:T1)  [unwired: 18 in]
            }
            frame Error {
              n160 = Unbundle By Name(w386) -> ("source"=w385:string)
              n161 = call-poly "CoreLib.data 2 byte array.vi"("string"=w385) -> ("byteArray out"=w384:T1)  [unwired: 18 in]
            }
          }
          n162 = Unbundle By Name(w374) -> ("code"=w379:i32)
          n163 = Bundle By Name(cluster=w378, "Data"=w368, "Error #"=w379) -> (w377:T2)
        }
        frame "SetDMode" {
          n164 = Unbundle By Name(w406) -> ("Data"=w399:T1)
          n165 = call-poly "CoreLib.byte array 2 data.vi"("byteArray"=w399) -> ("i32"=w397:i32, "error out"=w398:errorcluster)  [unwired: 16 in, 1 out]
          n166 = case shown="No Error" w398 {
            tunnel: [w415 w423] -> w404
            tunnel: w409 -> [w418 w423]
            tunnel: w408 -> [w416 w422]
            tunnel: [w417 w421] -> w403
            tunnel: w401 -> [_ w420]
            tunnel: w397 -> [w419 _]
            frame No Error {
              n167 = call "DG535.set D mode.vi"("i ref in"=w418, "mode"=w419, "error in"=w416) -> ("i ref out"=w415:refnum<vi>, "error out"=w417:errorcluster)  [unwired: 11 in]
            }
            frame Error {
              n168 = call "CoreLib.set data type mismatch.vi"("error in (no error)"=w422, "error source"=w420) -> ("error out"=w421:errorcluster)  [unwired: 17 in]
            }
          }
          n169 = call "BaseProcess.set event status.vi"("i ref in"=w404, "EventStatus"=w401, "error in (no error)"=w403) -> ("i ref out"=w400:refnum<vi>, "error out"=w402:errorcluster)  [unwired: 14 in, 1 out]
          n170 = case shown="Error" w402 {
            selector: w402 -> [_ w414]
            tunnel: [w410 w412] -> w396
            frame No Error {
              n171 = call-poly "CoreLib.data 2 byte array.vi"("string"="" ("source")) -> ("byteArray out"=w410:T1)  [unwired: 18 in]
            }
            frame Error {
              n172 = Unbundle By Name(w414) -> ("source"=w413:string)
              n173 = call-poly "CoreLib.data 2 byte array.vi"("string"=w413) -> ("byteArray out"=w412:T1)  [unwired: 18 in]
            }
          }
          n174 = Unbundle By Name(w402) -> ("code"=w407:i32)
          n175 = Bundle By Name(cluster=w406, "Data"=w396, "Error #"=w407) -> (w405:T2)
        }
        frame "SetCDMode" {
          n176 = Unbundle By Name(w434) -> ("Data"=w427:T1)
          n177 = call-poly "CoreLib.byte array 2 data.vi"("byteArray"=w427) -> ("i32"=w426:i32, "error out"=w425:errorcluster)  [unwired: 16 in, 1 out]
          n178 = case shown="No Error" w425 {
            tunnel: [w443 w451] -> w432
            tunnel: w437 -> [w446 w451]
            tunnel: w436 -> [w444 w450]
            tunnel: [w445 w449] -> w431
            tunnel: w429 -> [_ w448]
            tunnel: w426 -> [w447 _]
            frame No Error {
              n179 = call "DG535.set CD mode.vi"("i ref in"=w446, "mode"=w447, "error in"=w444) -> ("i ref out"=w443:refnum<vi>, "error out"=w445:errorcluster)  [unwired: 11 in]
            }
            frame Error {
              n180 = call "CoreLib.set data type mismatch.vi"("error in (no error)"=w450, "error source"=w448) -> ("error out"=w449:errorcluster)  [unwired: 17 in]
            }
          }
          n181 = call "BaseProcess.set event status.vi"("i ref in"=w432, "EventStatus"=w429, "error in (no error)"=w431) -> ("i ref out"=w428:refnum<vi>, "error out"=w430:errorcluster)  [unwired: 14 in, 1 out]
          n182 = case shown="Error" w430 {
            selector: w430 -> [_ w442]
            tunnel: [w438 w440] -> w424
            frame No Error {
              n183 = call-poly "CoreLib.data 2 byte array.vi"("string"="" ("source")) -> ("byteArray out"=w438:T1)  [unwired: 18 in]
            }
            frame Error {
              n184 = Unbundle By Name(w442) -> ("source"=w441:string)
              n185 = call-poly "CoreLib.data 2 byte array.vi"("string"=w441) -> ("byteArray out"=w440:T1)  [unwired: 18 in]
            }
          }
          n186 = Unbundle By Name(w430) -> ("code"=w435:i32)
          n187 = Bundle By Name(cluster=w434, "Data"=w424, "Error #"=w435) -> (w433:T2)
        }
        frame "SetABInversio" {
          n188 = Unbundle By Name(w466) -> ("Data"=w455:T1)
          n189 = call-poly "CoreLib.byte array 2 data.vi"("byteArray"=w455) -> ("i16"=w453:i16, "error out"=w454:errorcluster)  [unwired: 16 in, 1 out]
          n190 = Equal To 0?(x=w453) -> (x = 0?=w457:bool)
          n191 = Select(t=FALSE, s=w457, f=TRUE) -> (s? t:f=w456:bool)
          n192 = case shown="No Error" w454 {
            tunnel: [w475 w483] -> w464
            tunnel: w469 -> [w478 w483]
            tunnel: w468 -> [w476 w482]
            tunnel: [w477 w481] -> w463
            tunnel: w461 -> [_ w480]
            tunnel: w456 -> [w479 _]
            frame No Error {
              n193 = call "DG535.set AB inversion.vi"("i ref in"=w478, "inversion"=w479, "error in (no error)"=w476) -> ("i ref out"=w475:refnum<vi>, "error out"=w477:errorcluster)  [unwired: 11 in]
            }
            frame Error {
              n194 = call "CoreLib.set data type mismatch.vi"("error in (no error)"=w482, "error source"=w480) -> ("error out"=w481:errorcluster)  [unwired: 17 in]
            }
          }
          n195 = call "BaseProcess.set event status.vi"("i ref in"=w464, "EventStatus"=w461, "error in (no error)"=w463) -> ("i ref out"=w460:refnum<vi>, "error out"=w462:errorcluster)  [unwired: 14 in, 1 out]
          n196 = case shown="No Error" w462 {
            selector: w462 -> [_ w474]
            tunnel: [w470 w472] -> w452
            frame No Error {
              n197 = call-poly "CoreLib.data 2 byte array.vi"("string"="" ("source")) -> ("byteArray out"=w470:T1)  [unwired: 18 in]
            }
            frame Error {
              n198 = Unbundle By Name(w474) -> ("source"=w473:string)
              n199 = call-poly "CoreLib.data 2 byte array.vi"("string"=w473) -> ("byteArray out"=w472:T1)  [unwired: 18 in]
            }
          }
          n200 = Unbundle By Name(w462) -> ("code"=w467:i32)
          n201 = Bundle By Name(cluster=w466, "Data"=w452, "Error #"=w467) -> (w465:T2)
        }
        frame "SetCDInversion" {
          n202 = Unbundle By Name(w498) -> ("Data"=w488:T1)
          n203 = call-poly "CoreLib.byte array 2 data.vi"("byteArray"=w488) -> ("i16"=w487:i16, "error out"=w486:errorcluster)  [unwired: 16 in, 1 out]
          n204 = Equal To 0?(x=w487) -> (x = 0?=w489:bool)
          n205 = Select(t=FALSE, s=w489, f=TRUE) -> (s? t:f=w485:bool)
          n206 = case shown="No Error" w486 {
            tunnel: [w507 w515] -> w496
            tunnel: w501 -> [w510 w515]
            tunnel: w500 -> [w508 w514]
            tunnel: [w509 w513] -> w495
            tunnel: w493 -> [_ w512]
            tunnel: w485 -> [w511 _]
            frame No Error {
              n207 = call "DG535.set CD inversion.vi"("i ref in"=w510, "inversion"=w511, "error in (no error)"=w508) -> ("i ref out"=w507:refnum<vi>, "error out"=w509:errorcluster)  [unwired: 11 in]
            }
            frame Error {
              n208 = call "CoreLib.set data type mismatch.vi"("error in (no error)"=w514, "error source"=w512) -> ("error out"=w513:errorcluster)  [unwired: 17 in]
            }
          }
          n209 = call "BaseProcess.set event status.vi"("i ref in"=w496, "EventStatus"=w493, "error in (no error)"=w495) -> ("i ref out"=w492:refnum<vi>, "error out"=w494:errorcluster)  [unwired: 14 in, 1 out]
          n210 = case shown="Error" w494 {
            selector: w494 -> [_ w506]
            tunnel: [w502 w504] -> w484
            frame No Error {
              n211 = call-poly "CoreLib.data 2 byte array.vi"("string"="" ("source")) -> ("byteArray out"=w502:T1)  [unwired: 18 in]
            }
            frame Error {
              n212 = Unbundle By Name(w506) -> ("source"=w505:string)
              n213 = call-poly "CoreLib.data 2 byte array.vi"("string"=w505) -> ("byteArray out"=w504:T1)  [unwired: 18 in]
            }
          }
          n214 = Unbundle By Name(w494) -> ("code"=w499:i32)
          n215 = Bundle By Name(cluster=w498, "Data"=w484, "Error #"=w499) -> (w497:T2)
        }
        frame "SetT0Amplitude" {
          n216 = Unbundle By Name(w526) -> ("Data"=w519:T1)
          n217 = call-poly "CoreLib.byte array 2 data.vi"("byteArray"=w519) -> ("d64"=w518:dbl, "error out"=w517:errorcluster)  [unwired: 16 in, 1 out]
          n218 = case shown="No Error" w517 {
            tunnel: [w535 w543] -> w524
            tunnel: w529 -> [w538 w543]
            tunnel: w528 -> [w536 w542]
            tunnel: [w537 w541] -> w523
            tunnel: w521 -> [_ w540]
            tunnel: w518 -> [w539 _]
            frame No Error {
              n219 = call "DG535.set T0 amplitude.vi"("i ref in"=w538, "amplitude"=w539, "error in (no error)"=w536) -> ("i ref out"=w535:refnum<vi>, "error out"=w537:errorcluster)  [unwired: 11 in]
            }
            frame Error {
              n220 = call "CoreLib.set data type mismatch.vi"("error in (no error)"=w542, "error source"=w540) -> ("error out"=w541:errorcluster)  [unwired: 17 in]
            }
          }
          n221 = call "BaseProcess.set event status.vi"("i ref in"=w524, "EventStatus"=w521, "error in (no error)"=w523) -> ("i ref out"=w520:refnum<vi>, "error out"=w522:errorcluster)  [unwired: 14 in, 1 out]
          n222 = case shown="Error" w522 {
            selector: w522 -> [_ w534]
            tunnel: [w530 w532] -> w516
            frame No Error {
              n223 = call-poly "CoreLib.data 2 byte array.vi"("string"="" ("source")) -> ("byteArray out"=w530:T1)  [unwired: 18 in]
            }
            frame Error {
              n224 = Unbundle By Name(w534) -> ("source"=w533:string)
              n225 = call-poly "CoreLib.data 2 byte array.vi"("string"=w533) -> ("byteArray out"=w532:T1)  [unwired: 18 in]
            }
          }
          n226 = Unbundle By Name(w522) -> ("code"=w527:i32)
          n227 = Bundle By Name(cluster=w526, "Data"=w516, "Error #"=w527) -> (w525:T2)
        }
        frame "SetAAmplitude" {
          n228 = Unbundle By Name(w554) -> ("Data"=w547:T1)
          n229 = call-poly "CoreLib.byte array 2 data.vi"("byteArray"=w547) -> ("d64"=w545:dbl, "error out"=w546:errorcluster)  [unwired: 16 in, 1 out]
          n230 = case shown="No Error" w546 {
            tunnel: [w563 w571] -> w552
            tunnel: w557 -> [w566 w571]
            tunnel: w556 -> [w564 w570]
            tunnel: [w565 w569] -> w551
            tunnel: w549 -> [_ w568]
            tunnel: w545 -> [w567 _]
            frame No Error {
              n231 = call "DG535.set A amplitude.vi"("i ref in"=w566, "amplitude"=w567, "error in (no error)"=w564) -> ("i ref out"=w563:refnum<vi>, "error out"=w565:errorcluster)  [unwired: 11 in]
            }
            frame Error {
              n232 = call "CoreLib.set data type mismatch.vi"("error in (no error)"=w570, "error source"=w568) -> ("error out"=w569:errorcluster)  [unwired: 17 in]
            }
          }
          n233 = call "BaseProcess.set event status.vi"("i ref in"=w552, "EventStatus"=w549, "error in (no error)"=w551) -> ("i ref out"=w548:refnum<vi>, "error out"=w550:errorcluster)  [unwired: 14 in, 1 out]
          n234 = case shown="Error" w550 {
            selector: w550 -> [_ w562]
            tunnel: [w558 w560] -> w544
            frame No Error {
              n235 = call-poly "CoreLib.data 2 byte array.vi"("string"="" ("source")) -> ("byteArray out"=w558:T1)  [unwired: 18 in]
            }
            frame Error {
              n236 = Unbundle By Name(w562) -> ("source"=w561:string)
              n237 = call-poly "CoreLib.data 2 byte array.vi"("string"=w561) -> ("byteArray out"=w560:T1)  [unwired: 18 in]
            }
          }
          n238 = Unbundle By Name(w550) -> ("code"=w555:i32)
          n239 = Bundle By Name(cluster=w554, "Data"=w544, "Error #"=w555) -> (w553:T2)
        }
        frame "SetBAmplitude" {
          n240 = Unbundle By Name(w582) -> ("Data"=w575:T1)
          n241 = call-poly "CoreLib.byte array 2 data.vi"("byteArray"=w575) -> ("d64"=w573:dbl, "error out"=w574:errorcluster)  [unwired: 16 in, 1 out]
          n242 = case shown="No Error" w574 {
            tunnel: [w591 w599] -> w580
            tunnel: w585 -> [w594 w599]
            tunnel: w584 -> [w592 w598]
            tunnel: [w593 w597] -> w579
            tunnel: w577 -> [_ w596]
            tunnel: w573 -> [w595 _]
            frame No Error {
              n243 = call "DG535.set B amplitude.vi"("i ref in"=w594, "amplitude"=w595, "error in (no error)"=w592) -> ("i ref out"=w591:refnum<vi>, "error out"=w593:errorcluster)  [unwired: 11 in]
            }
            frame Error {
              n244 = call "CoreLib.set data type mismatch.vi"("error in (no error)"=w598, "error source"=w596) -> ("error out"=w597:errorcluster)  [unwired: 17 in]
            }
          }
          n245 = call "BaseProcess.set event status.vi"("i ref in"=w580, "EventStatus"=w577, "error in (no error)"=w579) -> ("i ref out"=w576:refnum<vi>, "error out"=w578:errorcluster)  [unwired: 14 in, 1 out]
          n246 = case shown="No Error" w578 {
            selector: w578 -> [_ w590]
            tunnel: [w586 w588] -> w572
            frame No Error {
              n247 = call-poly "CoreLib.data 2 byte array.vi"("string"="" ("source")) -> ("byteArray out"=w586:T1)  [unwired: 18 in]
            }
            frame Error {
              n248 = Unbundle By Name(w590) -> ("source"=w589:string)
              n249 = call-poly "CoreLib.data 2 byte array.vi"("string"=w589) -> ("byteArray out"=w588:T1)  [unwired: 18 in]
            }
          }
          n250 = Unbundle By Name(w578) -> ("code"=w583:i32)
          n251 = Bundle By Name(cluster=w582, "Data"=w572, "Error #"=w583) -> (w581:T2)
        }
        frame "SetABAmplitude" {
          n252 = Unbundle By Name(w610) -> ("Data"=w603:T1)
          n253 = call-poly "CoreLib.byte array 2 data.vi"("byteArray"=w603) -> ("d64"=w601:dbl, "error out"=w602:errorcluster)  [unwired: 16 in, 1 out]
          n254 = case shown="No Error" w602 {
            tunnel: [w619 w627] -> w608
            tunnel: w613 -> [w622 w627]
            tunnel: w612 -> [w620 w626]
            tunnel: [w621 w625] -> w607
            tunnel: w605 -> [_ w624]
            tunnel: w601 -> [w623 _]
            frame No Error {
              n255 = call "DG535.set AB amplitude.vi"("i ref in"=w622, "amplitude"=w623, "error in (no error)"=w620) -> ("i ref out"=w619:refnum<vi>, "error out"=w621:errorcluster)  [unwired: 11 in]
            }
            frame Error {
              n256 = call "CoreLib.set data type mismatch.vi"("error in (no error)"=w626, "error source"=w624) -> ("error out"=w625:errorcluster)  [unwired: 17 in]
            }
          }
          n257 = call "BaseProcess.set event status.vi"("i ref in"=w608, "EventStatus"=w605, "error in (no error)"=w607) -> ("i ref out"=w604:refnum<vi>, "error out"=w606:errorcluster)  [unwired: 14 in, 1 out]
          n258 = case shown="Error" w606 {
            selector: w606 -> [_ w618]
            tunnel: [w614 w616] -> w600
            frame No Error {
              n259 = call-poly "CoreLib.data 2 byte array.vi"("string"="" ("source")) -> ("byteArray out"=w614:T1)  [unwired: 18 in]
            }
            frame Error {
              n260 = Unbundle By Name(w618) -> ("source"=w617:string)
              n261 = call-poly "CoreLib.data 2 byte array.vi"("string"=w617) -> ("byteArray out"=w616:T1)  [unwired: 18 in]
            }
          }
          n262 = Unbundle By Name(w606) -> ("code"=w611:i32)
          n263 = Bundle By Name(cluster=w610, "Data"=w600, "Error #"=w611) -> (w609:T2)
        }
        frame "SetCAmplitude" {
          n264 = Unbundle By Name(w638) -> ("Data"=w631:T1)
          n265 = call-poly "CoreLib.byte array 2 data.vi"("byteArray"=w631) -> ("d64"=w629:dbl, "error out"=w630:errorcluster)  [unwired: 16 in, 1 out]
          n266 = case shown="No Error" w630 {
            tunnel: [w647 w655] -> w636
            tunnel: w641 -> [w650 w655]
            tunnel: w640 -> [w648 w654]
            tunnel: [w649 w653] -> w635
            tunnel: w633 -> [_ w652]
            tunnel: w629 -> [w651 _]
            frame No Error {
              n267 = call "DG535.set C amplitude.vi"("i ref in"=w650, "amplitude"=w651, "error in (no error)"=w648) -> ("i ref out"=w647:refnum<vi>, "error out"=w649:errorcluster)  [unwired: 11 in]
            }
            frame Error {
              n268 = call "CoreLib.set data type mismatch.vi"("error in (no error)"=w654, "error source"=w652) -> ("error out"=w653:errorcluster)  [unwired: 17 in]
            }
          }
          n269 = call "BaseProcess.set event status.vi"("i ref in"=w636, "EventStatus"=w633, "error in (no error)"=w635) -> ("i ref out"=w632:refnum<vi>, "error out"=w634:errorcluster)  [unwired: 14 in, 1 out]
          n270 = case shown="Error" w634 {
            selector: w634 -> [_ w646]
            tunnel: [w642 w644] -> w628
            frame No Error {
              n271 = call-poly "CoreLib.data 2 byte array.vi"("string"="" ("source")) -> ("byteArray out"=w642:T1)  [unwired: 18 in]
            }
            frame Error {
              n272 = Unbundle By Name(w646) -> ("source"=w645:string)
              n273 = call-poly "CoreLib.data 2 byte array.vi"("string"=w645) -> ("byteArray out"=w644:T1)  [unwired: 18 in]
            }
          }
          n274 = Unbundle By Name(w634) -> ("code"=w639:i32)
          n275 = Bundle By Name(cluster=w638, "Data"=w628, "Error #"=w639) -> (w637:T2)
        }
        frame "SetDAmplitude" {
          n276 = Unbundle By Name(w666) -> ("Data"=w659:T1)
          n277 = call-poly "CoreLib.byte array 2 data.vi"("byteArray"=w659) -> ("d64"=w658:dbl, "error out"=w657:errorcluster)  [unwired: 16 in, 1 out]
          n278 = case shown="No Error" w657 {
            tunnel: [w675 w683] -> w664
            tunnel: w669 -> [w678 w683]
            tunnel: w668 -> [w676 w682]
            tunnel: [w677 w681] -> w663
            tunnel: w661 -> [_ w680]
            tunnel: w658 -> [w679 _]
            frame No Error {
              n279 = call "DG535.set D amplitude.vi"("i ref in"=w678, "amplitude"=w679, "error in (no error)"=w676) -> ("i ref out"=w675:refnum<vi>, "error out"=w677:errorcluster)  [unwired: 11 in]
            }
            frame Error {
              n280 = call "CoreLib.set data type mismatch.vi"("error in (no error)"=w682, "error source"=w680) -> ("error out"=w681:errorcluster)  [unwired: 17 in]
            }
          }
          n281 = call "BaseProcess.set event status.vi"("i ref in"=w664, "EventStatus"=w661, "error in (no error)"=w663) -> ("i ref out"=w660:refnum<vi>, "error out"=w662:errorcluster)  [unwired: 14 in, 1 out]
          n282 = case shown="Error" w662 {
            selector: w662 -> [_ w674]
            tunnel: [w670 w672] -> w656
            frame No Error {
              n283 = call-poly "CoreLib.data 2 byte array.vi"("string"="" ("source")) -> ("byteArray out"=w670:T1)  [unwired: 18 in]
            }
            frame Error {
              n284 = Unbundle By Name(w674) -> ("source"=w673:string)
              n285 = call-poly "CoreLib.data 2 byte array.vi"("string"=w673) -> ("byteArray out"=w672:T1)  [unwired: 18 in]
            }
          }
          n286 = Unbundle By Name(w662) -> ("code"=w667:i32)
          n287 = Bundle By Name(cluster=w666, "Data"=w656, "Error #"=w667) -> (w665:T2)
        }
        frame "SetCDAmplitude" {
          n288 = Unbundle By Name(w694) -> ("Data"=w687:T1)
          n289 = call-poly "CoreLib.byte array 2 data.vi"("byteArray"=w687) -> ("d64"=w685:dbl, "error out"=w686:errorcluster)  [unwired: 16 in, 1 out]
          n290 = case shown="No Error" w686 {
            tunnel: [w703 w711] -> w692
            tunnel: w697 -> [w706 w711]
            tunnel: w696 -> [w704 w710]
            tunnel: [w705 w709] -> w691
            tunnel: w689 -> [_ w708]
            tunnel: w685 -> [w707 _]
            frame No Error {
              n291 = call "DG535.set CD amplitude.vi"("i ref in"=w706, "amplitude"=w707, "error in (no error)"=w704) -> ("i ref out"=w703:refnum<vi>, "error out"=w705:errorcluster)  [unwired: 11 in]
            }
            frame Error {
              n292 = call "CoreLib.set data type mismatch.vi"("error in (no error)"=w710, "error source"=w708) -> ("error out"=w709:errorcluster)  [unwired: 17 in]
            }
          }
          n293 = call "BaseProcess.set event status.vi"("i ref in"=w692, "EventStatus"=w689, "error in (no error)"=w691) -> ("i ref out"=w688:refnum<vi>, "error out"=w690:errorcluster)  [unwired: 14 in, 1 out]
          n294 = case shown="Error" w690 {
            selector: w690 -> [_ w702]
            tunnel: [w698 w700] -> w684
            frame No Error {
              n295 = call-poly "CoreLib.data 2 byte array.vi"("string"="" ("source")) -> ("byteArray out"=w698:T1)  [unwired: 18 in]
            }
            frame Error {
              n296 = Unbundle By Name(w702) -> ("source"=w701:string)
              n297 = call-poly "CoreLib.data 2 byte array.vi"("string"=w701) -> ("byteArray out"=w700:T1)  [unwired: 18 in]
            }
          }
          n298 = Unbundle By Name(w690) -> ("code"=w695:i32)
          n299 = Bundle By Name(cluster=w694, "Data"=w684, "Error #"=w695) -> (w693:T2)
        }
        frame "SetT0Offset" {
          n300 = Unbundle By Name(w722) -> ("Data"=w715:T1)
          n301 = call-poly "CoreLib.byte array 2 data.vi"("byteArray"=w715) -> ("d64"=w713:dbl, "error out"=w714:errorcluster)  [unwired: 16 in, 1 out]
          n302 = case shown="No Error" w714 {
            tunnel: [w731 w739] -> w720
            tunnel: w725 -> [w734 w739]
            tunnel: w724 -> [w732 w738]
            tunnel: [w733 w737] -> w719
            tunnel: w717 -> [_ w736]
            tunnel: w713 -> [w735 _]
            frame No Error {
              n303 = call "DG535.set T0 offset.vi"("i ref in"=w734, "offset"=w735, "error in (no error)"=w732) -> ("i ref out"=w731:refnum<vi>, "error out"=w733:errorcluster)  [unwired: 11 in]
            }
            frame Error {
              n304 = call "CoreLib.set data type mismatch.vi"("error in (no error)"=w738, "error source"=w736) -> ("error out"=w737:errorcluster)  [unwired: 17 in]
            }
          }
          n305 = call "BaseProcess.set event status.vi"("i ref in"=w720, "EventStatus"=w717, "error in (no error)"=w719) -> ("i ref out"=w716:refnum<vi>, "error out"=w718:errorcluster)  [unwired: 14 in, 1 out]
          n306 = case shown="No Error" w718 {
            selector: w718 -> [_ w730]
            tunnel: [w726 w728] -> w712
            frame No Error {
              n307 = call-poly "CoreLib.data 2 byte array.vi"("string"="" ("source")) -> ("byteArray out"=w726:T1)  [unwired: 18 in]
            }
            frame Error {
              n308 = Unbundle By Name(w730) -> ("source"=w729:string)
              n309 = call-poly "CoreLib.data 2 byte array.vi"("string"=w729) -> ("byteArray out"=w728:T1)  [unwired: 18 in]
            }
          }
          n310 = Unbundle By Name(w718) -> ("code"=w723:i32)
          n311 = Bundle By Name(cluster=w722, "Data"=w712, "Error #"=w723) -> (w721:T2)
        }
        frame "SetAOffset" {
          n312 = Unbundle By Name(w750) -> ("Data"=w743:T1)
          n313 = call-poly "CoreLib.byte array 2 data.vi"("byteArray"=w743) -> ("d64"=w742:dbl, "error out"=w741:errorcluster)  [unwired: 16 in, 1 out]
          n314 = case shown="No Error" w741 {
            tunnel: [w759 w767] -> w748
            tunnel: w753 -> [w762 w767]
            tunnel: w752 -> [w760 w766]
            tunnel: [w761 w765] -> w747
            tunnel: w745 -> [_ w764]
            tunnel: w742 -> [w763 _]
            frame No Error {
              n315 = call "DG535.set A offset.vi"("i ref in"=w762, "offset"=w763, "error in (no error)"=w760) -> ("i ref out"=w759:refnum<vi>, "error out"=w761:errorcluster)  [unwired: 11 in]
            }
            frame Error {
              n316 = call "CoreLib.set data type mismatch.vi"("error in (no error)"=w766, "error source"=w764) -> ("error out"=w765:errorcluster)  [unwired: 17 in]
            }
          }
          n317 = call "BaseProcess.set event status.vi"("i ref in"=w748, "EventStatus"=w745, "error in (no error)"=w747) -> ("i ref out"=w744:refnum<vi>, "error out"=w746:errorcluster)  [unwired: 14 in, 1 out]
          n318 = case shown="No Error" w746 {
            selector: w746 -> [_ w758]
            tunnel: [w754 w756] -> w740
            frame No Error {
              n319 = call-poly "CoreLib.data 2 byte array.vi"("string"="" ("source")) -> ("byteArray out"=w754:T1)  [unwired: 18 in]
            }
            frame Error {
              n320 = Unbundle By Name(w758) -> ("source"=w757:string)
              n321 = call-poly "CoreLib.data 2 byte array.vi"("string"=w757) -> ("byteArray out"=w756:T1)  [unwired: 18 in]
            }
          }
          n322 = Unbundle By Name(w746) -> ("code"=w751:i32)
          n323 = Bundle By Name(cluster=w750, "Data"=w740, "Error #"=w751) -> (w749:T2)
        }
        frame "SetBOffset" {
          n324 = Unbundle By Name(w778) -> ("Data"=w771:T1)
          n325 = call-poly "CoreLib.byte array 2 data.vi"("byteArray"=w771) -> ("d64"=w770:dbl, "error out"=w769:errorcluster)  [unwired: 16 in, 1 out]
          n326 = case shown="No Error" w769 {
            tunnel: [w787 w795] -> w776
            tunnel: w781 -> [w790 w795]
            tunnel: w780 -> [w788 w794]
            tunnel: [w789 w793] -> w775
            tunnel: w773 -> [_ w792]
            tunnel: w770 -> [w791 _]
            frame No Error {
              n327 = call "DG535.set B offset.vi"("i ref in"=w790, "offset"=w791, "error in (no error)"=w788) -> ("i ref out"=w787:refnum<vi>, "error out"=w789:errorcluster)  [unwired: 11 in]
            }
            frame Error {
              n328 = call "CoreLib.set data type mismatch.vi"("error in (no error)"=w794, "error source"=w792) -> ("error out"=w793:errorcluster)  [unwired: 17 in]
            }
          }
          n329 = call "BaseProcess.set event status.vi"("i ref in"=w776, "EventStatus"=w773, "error in (no error)"=w775) -> ("i ref out"=w772:refnum<vi>, "error out"=w774:errorcluster)  [unwired: 14 in, 1 out]
          n330 = case shown="Error" w774 {
            selector: w774 -> [_ w786]
            tunnel: [w782 w784] -> w768
            frame No Error {
              n331 = call-poly "CoreLib.data 2 byte array.vi"("string"="" ("source")) -> ("byteArray out"=w782:T1)  [unwired: 18 in]
            }
            frame Error {
              n332 = Unbundle By Name(w786) -> ("source"=w785:string)
              n333 = call-poly "CoreLib.data 2 byte array.vi"("string"=w785) -> ("byteArray out"=w784:T1)  [unwired: 18 in]
            }
          }
          n334 = Unbundle By Name(w774) -> ("code"=w779:i32)
          n335 = Bundle By Name(cluster=w778, "Data"=w768, "Error #"=w779) -> (w777:T2)
        }
        frame "SetABOffset" {
          n336 = Unbundle By Name(w806) -> ("Data"=w799:T1)
          n337 = call-poly "CoreLib.byte array 2 data.vi"("byteArray"=w799) -> ("d64"=w797:dbl, "error out"=w798:errorcluster)  [unwired: 16 in, 1 out]
          n338 = case shown="No Error" w798 {
            tunnel: [w815 w823] -> w804
            tunnel: w809 -> [w818 w823]
            tunnel: w808 -> [w816 w822]
            tunnel: [w817 w821] -> w803
            tunnel: w801 -> [_ w820]
            tunnel: w797 -> [w819 _]
            frame No Error {
              n339 = call "DG535.set AB offset.vi"("i ref in"=w818, "offset"=w819, "error in (no error)"=w816) -> ("i ref out"=w815:refnum<vi>, "error out"=w817:errorcluster)  [unwired: 11 in]
            }
            frame Error {
              n340 = call "CoreLib.set data type mismatch.vi"("error in (no error)"=w822, "error source"=w820) -> ("error out"=w821:errorcluster)  [unwired: 17 in]
            }
          }
          n341 = call "BaseProcess.set event status.vi"("i ref in"=w804, "EventStatus"=w801, "error in (no error)"=w803) -> ("i ref out"=w800:refnum<vi>, "error out"=w802:errorcluster)  [unwired: 14 in, 1 out]
          n342 = case shown="Error" w802 {
            selector: w802 -> [_ w814]
            tunnel: [w810 w812] -> w796
            frame No Error {
              n343 = call-poly "CoreLib.data 2 byte array.vi"("string"="" ("source")) -> ("byteArray out"=w810:T1)  [unwired: 18 in]
            }
            frame Error {
              n344 = Unbundle By Name(w814) -> ("source"=w813:string)
              n345 = call-poly "CoreLib.data 2 byte array.vi"("string"=w813) -> ("byteArray out"=w812:T1)  [unwired: 18 in]
            }
          }
          n346 = Unbundle By Name(w802) -> ("code"=w807:i32)
          n347 = Bundle By Name(cluster=w806, "Data"=w796, "Error #"=w807) -> (w805:T2)
        }
        frame "SetCOffset" {
          n348 = Unbundle By Name(w834) -> ("Data"=w827:T1)
          n349 = call-poly "CoreLib.byte array 2 data.vi"("byteArray"=w827) -> ("d64"=w826:dbl, "error out"=w825:errorcluster)  [unwired: 16 in, 1 out]
          n350 = case shown="No Error" w825 {
            tunnel: [w843 w851] -> w832
            tunnel: w837 -> [w846 w851]
            tunnel: w836 -> [w844 w850]
            tunnel: [w845 w849] -> w831
            tunnel: w829 -> [_ w848]
            tunnel: w826 -> [w847 _]
            frame No Error {
              n351 = call "DG535.set C offset.vi"("i ref in"=w846, "offset"=w847, "error in (no error)"=w844) -> ("i ref out"=w843:refnum<vi>, "error out"=w845:errorcluster)  [unwired: 11 in]
            }
            frame Error {
              n352 = call "CoreLib.set data type mismatch.vi"("error in (no error)"=w850, "error source"=w848) -> ("error out"=w849:errorcluster)  [unwired: 17 in]
            }
          }
          n353 = call "BaseProcess.set event status.vi"("i ref in"=w832, "EventStatus"=w829, "error in (no error)"=w831) -> ("i ref out"=w828:refnum<vi>, "error out"=w830:errorcluster)  [unwired: 14 in, 1 out]
          n354 = case shown="Error" w830 {
            selector: w830 -> [_ w842]
            tunnel: [w838 w840] -> w824
            frame No Error {
              n355 = call-poly "CoreLib.data 2 byte array.vi"("string"="" ("source")) -> ("byteArray out"=w838:T1)  [unwired: 18 in]
            }
            frame Error {
              n356 = Unbundle By Name(w842) -> ("source"=w841:string)
              n357 = call-poly "CoreLib.data 2 byte array.vi"("string"=w841) -> ("byteArray out"=w840:T1)  [unwired: 18 in]
            }
          }
          n358 = Unbundle By Name(w830) -> ("code"=w835:i32)
          n359 = Bundle By Name(cluster=w834, "Data"=w824, "Error #"=w835) -> (w833:T2)
        }
        frame "SetDOffset" {
          n360 = Unbundle By Name(w862) -> ("Data"=w855:T1)
          n361 = call-poly "CoreLib.byte array 2 data.vi"("byteArray"=w855) -> ("d64"=w854:dbl, "error out"=w853:errorcluster)  [unwired: 16 in, 1 out]
          n362 = case shown="No Error" w853 {
            tunnel: [w871 w879] -> w860
            tunnel: w865 -> [w874 w879]
            tunnel: w864 -> [w872 w878]
            tunnel: [w873 w877] -> w859
            tunnel: w857 -> [_ w876]
            tunnel: w854 -> [w875 _]
            frame No Error {
              n363 = call "DG535.set D offset.vi"("i ref in"=w874, "offset"=w875, "error in (no error)"=w872) -> ("i ref out"=w871:refnum<vi>, "error out"=w873:errorcluster)  [unwired: 11 in]
            }
            frame Error {
              n364 = call "CoreLib.set data type mismatch.vi"("error in (no error)"=w878, "error source"=w876) -> ("error out"=w877:errorcluster)  [unwired: 17 in]
            }
          }
          n365 = call "BaseProcess.set event status.vi"("i ref in"=w860, "EventStatus"=w857, "error in (no error)"=w859) -> ("i ref out"=w856:refnum<vi>, "error out"=w858:errorcluster)  [unwired: 14 in, 1 out]
          n366 = case shown="Error" w858 {
            selector: w858 -> [_ w870]
            tunnel: [w866 w868] -> w852
            frame No Error {
              n367 = call-poly "CoreLib.data 2 byte array.vi"("string"="" ("source")) -> ("byteArray out"=w866:T1)  [unwired: 18 in]
            }
            frame Error {
              n368 = Unbundle By Name(w870) -> ("source"=w869:string)
              n369 = call-poly "CoreLib.data 2 byte array.vi"("string"=w869) -> ("byteArray out"=w868:T1)  [unwired: 18 in]
            }
          }
          n370 = Unbundle By Name(w858) -> ("code"=w863:i32)
          n371 = Bundle By Name(cluster=w862, "Data"=w852, "Error #"=w863) -> (w861:T2)
        }
        frame "SetCDOffset" {
          n372 = Unbundle By Name(w890) -> ("Data"=w883:T1)
          n373 = call-poly "CoreLib.byte array 2 data.vi"("byteArray"=w883) -> ("d64"=w882:dbl, "error out"=w881:errorcluster)  [unwired: 16 in, 1 out]
          n374 = case shown="No Error" w881 {
            tunnel: [w899 w907] -> w888
            tunnel: w893 -> [w902 w907]
            tunnel: w892 -> [w900 w906]
            tunnel: [w901 w905] -> w887
            tunnel: w885 -> [_ w904]
            tunnel: w882 -> [w903 _]
            frame No Error {
              n375 = call "DG535.set CD offset.vi"("i ref in"=w902, "offset"=w903, "error in (no error)"=w900) -> ("i ref out"=w899:refnum<vi>, "error out"=w901:errorcluster)  [unwired: 11 in]
            }
            frame Error {
              n376 = call "CoreLib.set data type mismatch.vi"("error in (no error)"=w906, "error source"=w904) -> ("error out"=w905:errorcluster)  [unwired: 17 in]
            }
          }
          n377 = call "BaseProcess.set event status.vi"("i ref in"=w888, "EventStatus"=w885, "error in (no error)"=w887) -> ("i ref out"=w884:refnum<vi>, "error out"=w886:errorcluster)  [unwired: 14 in, 1 out]
          n378 = case shown="Error" w886 {
            selector: w886 -> [_ w898]
            tunnel: [w894 w896] -> w880
            frame No Error {
              n379 = call-poly "CoreLib.data 2 byte array.vi"("string"="" ("source")) -> ("byteArray out"=w894:T1)  [unwired: 18 in]
            }
            frame Error {
              n380 = Unbundle By Name(w898) -> ("source"=w897:string)
              n381 = call-poly "CoreLib.data 2 byte array.vi"("string"=w897) -> ("byteArray out"=w896:T1)  [unwired: 18 in]
            }
          }
          n382 = Unbundle By Name(w886) -> ("code"=w891:i32)
          n383 = Bundle By Name(cluster=w890, "Data"=w880, "Error #"=w891) -> (w889:T2)
        }
        frame "SetT0Load" {
          n384 = Unbundle By Name(w922) -> ("Data"=w912:T1)
          n385 = call-poly "CoreLib.byte array 2 data.vi"("byteArray"=w912) -> ("i16"=w911:i16, "error out"=w910:errorcluster)  [unwired: 16 in, 1 out]
          n386 = Equal To 0?(x=w911) -> (x = 0?=w913:bool)
          n387 = Select(t=FALSE, s=w913, f=TRUE) -> (s? t:f=w909:bool)
          n388 = case shown="No Error" w910 {
            tunnel: [w931 w939] -> w920
            tunnel: w925 -> [w934 w939]
            tunnel: w924 -> [w932 w938]
            tunnel: [w933 w937] -> w919
            tunnel: w917 -> [_ w936]
            tunnel: w909 -> [w935 _]
            frame No Error {
              n389 = call "DG535.set T0 load.vi"("i ref in"=w934, "load"=w935, "error in (no error)"=w932) -> ("i ref out"=w931:refnum<vi>, "error out"=w933:errorcluster)  [unwired: 11 in]
            }
            frame Error {
              n390 = call "CoreLib.set data type mismatch.vi"("error in (no error)"=w938, "error source"=w936) -> ("error out"=w937:errorcluster)  [unwired: 17 in]
            }
          }
          n391 = call "BaseProcess.set event status.vi"("i ref in"=w920, "EventStatus"=w917, "error in (no error)"=w919) -> ("i ref out"=w916:refnum<vi>, "error out"=w918:errorcluster)  [unwired: 14 in, 1 out]
          n392 = case shown="Error" w918 {
            selector: w918 -> [_ w930]
            tunnel: [w926 w928] -> w908
            frame No Error {
              n393 = call-poly "CoreLib.data 2 byte array.vi"("string"="" ("source")) -> ("byteArray out"=w926:T1)  [unwired: 18 in]
            }
            frame Error {
              n394 = Unbundle By Name(w930) -> ("source"=w929:string)
              n395 = call-poly "CoreLib.data 2 byte array.vi"("string"=w929) -> ("byteArray out"=w928:T1)  [unwired: 18 in]
            }
          }
          n396 = Unbundle By Name(w918) -> ("code"=w923:i32)
          n397 = Bundle By Name(cluster=w922, "Data"=w908, "Error #"=w923) -> (w921:T2)
        }
        frame "SetALoad" {
          n398 = Unbundle By Name(w954) -> ("Data"=w944:T1)
          n399 = call-poly "CoreLib.byte array 2 data.vi"("byteArray"=w944) -> ("i16"=w943:i16, "error out"=w942:errorcluster)  [unwired: 16 in, 1 out]
          n400 = Equal To 0?(x=w943) -> (x = 0?=w945:bool)
          n401 = Select(t=FALSE, s=w945, f=TRUE) -> (s? t:f=w941:bool)
          n402 = case shown="No Error" w942 {
            tunnel: [w963 w971] -> w952
            tunnel: w957 -> [w966 w971]
            tunnel: w956 -> [w964 w970]
            tunnel: [w965 w969] -> w951
            tunnel: w949 -> [_ w968]
            tunnel: w941 -> [w967 _]
            frame No Error {
              n403 = call "DG535.set A load.vi"("i ref in"=w966, "load"=w967, "error in (no error)"=w964) -> ("i ref out"=w963:refnum<vi>, "error out"=w965:errorcluster)  [unwired: 11 in]
            }
            frame Error {
              n404 = call "CoreLib.set data type mismatch.vi"("error in (no error)"=w970, "error source"=w968) -> ("error out"=w969:errorcluster)  [unwired: 17 in]
            }
          }
          n405 = call "BaseProcess.set event status.vi"("i ref in"=w952, "EventStatus"=w949, "error in (no error)"=w951) -> ("i ref out"=w948:refnum<vi>, "error out"=w950:errorcluster)  [unwired: 14 in, 1 out]
          n406 = case shown="No Error" w950 {
            selector: w950 -> [_ w962]
            tunnel: [w958 w960] -> w940
            frame No Error {
              n407 = call-poly "CoreLib.data 2 byte array.vi"("string"="" ("source")) -> ("byteArray out"=w958:T1)  [unwired: 18 in]
            }
            frame Error {
              n408 = Unbundle By Name(w962) -> ("source"=w961:string)
              n409 = call-poly "CoreLib.data 2 byte array.vi"("string"=w961) -> ("byteArray out"=w960:T1)  [unwired: 18 in]
            }
          }
          n410 = Unbundle By Name(w950) -> ("code"=w955:i32)
          n411 = Bundle By Name(cluster=w954, "Data"=w940, "Error #"=w955) -> (w953:T2)
        }
        frame "SetBLoad" {
          n412 = Unbundle By Name(w986) -> ("Data"=w976:T1)
          n413 = call-poly "CoreLib.byte array 2 data.vi"("byteArray"=w976) -> ("i16"=w975:i16, "error out"=w974:errorcluster)  [unwired: 16 in, 1 out]
          n414 = Equal To 0?(x=w975) -> (x = 0?=w977:bool)
          n415 = Select(t=FALSE, s=w977, f=TRUE) -> (s? t:f=w973:bool)
          n416 = case shown="No Error" w974 {
            tunnel: [w995 w1003] -> w984
            tunnel: w989 -> [w998 w1003]
            tunnel: w988 -> [w996 w1002]
            tunnel: [w997 w1001] -> w983
            tunnel: w981 -> [_ w1000]
            tunnel: w973 -> [w999 _]
            frame No Error {
              n417 = call "DG535.set B load.vi"("i ref in"=w998, "load"=w999, "error in (no error)"=w996) -> ("i ref out"=w995:refnum<vi>, "error out"=w997:errorcluster)  [unwired: 11 in]
            }
            frame Error {
              n418 = call "CoreLib.set data type mismatch.vi"("error in (no error)"=w1002, "error source"=w1000) -> ("error out"=w1001:errorcluster)  [unwired: 17 in]
            }
          }
          n419 = call "BaseProcess.set event status.vi"("i ref in"=w984, "EventStatus"=w981, "error in (no error)"=w983) -> ("i ref out"=w980:refnum<vi>, "error out"=w982:errorcluster)  [unwired: 14 in, 1 out]
          n420 = case shown="Error" w982 {
            selector: w982 -> [_ w994]
            tunnel: [w990 w993] -> w972
            frame No Error {
              n421 = call-poly "CoreLib.data 2 byte array.vi"("string"="" ("source")) -> ("byteArray out"=w990:T1)  [unwired: 18 in]
            }
            frame Error {
              n422 = Unbundle By Name(w994) -> ("source"=w992:string)
              n423 = call-poly "CoreLib.data 2 byte array.vi"("string"=w992) -> ("byteArray out"=w993:T1)  [unwired: 18 in]
            }
          }
          n424 = Unbundle By Name(w982) -> ("code"=w987:i32)
          n425 = Bundle By Name(cluster=w986, "Data"=w972, "Error #"=w987) -> (w985:T2)
        }
        frame "SetABLoad" {
          n426 = Unbundle By Name(w1018) -> ("Data"=w1011:T1)
          n427 = call-poly "CoreLib.byte array 2 data.vi"("byteArray"=w1011) -> ("i16"=w1007:i16, "error out"=w1006:errorcluster)  [unwired: 16 in, 1 out]
          n428 = Equal To 0?(x=w1007) -> (x = 0?=w1008:bool)
          n429 = Select(t=FALSE, s=w1008, f=TRUE) -> (s? t:f=w1005:bool)
          n430 = case shown="No Error" w1006 {
            tunnel: [w1027 w1035] -> w1016
            tunnel: w1021 -> [w1030 w1035]
            tunnel: w1020 -> [w1028 w1034]
            tunnel: [w1029 w1033] -> w1015
            tunnel: w1013 -> [_ w1032]
            tunnel: w1005 -> [w1031 _]
            frame No Error {
              n431 = call "DG535.set AB load.vi"("i ref in"=w1030, "load"=w1031, "error in (no error)"=w1028) -> ("i ref out"=w1027:refnum<vi>, "error out"=w1029:errorcluster)  [unwired: 11 in]
            }
            frame Error {
              n432 = call "CoreLib.set data type mismatch.vi"("error in (no error)"=w1034, "error source"=w1032) -> ("error out"=w1033:errorcluster)  [unwired: 17 in]
            }
          }
          n433 = call "BaseProcess.set event status.vi"("i ref in"=w1016, "EventStatus"=w1013, "error in (no error)"=w1015) -> ("i ref out"=w1012:refnum<vi>, "error out"=w1014:errorcluster)  [unwired: 14 in, 1 out]
          n434 = case shown="Error" w1014 {
            selector: w1014 -> [_ w1026]
            tunnel: [w1022 w1024] -> w1004
            frame No Error {
              n435 = call-poly "CoreLib.data 2 byte array.vi"("string"="" ("source")) -> ("byteArray out"=w1022:T1)  [unwired: 18 in]
            }
            frame Error {
              n436 = Unbundle By Name(w1026) -> ("source"=w1025:string)
              n437 = call-poly "CoreLib.data 2 byte array.vi"("string"=w1025) -> ("byteArray out"=w1024:T1)  [unwired: 18 in]
            }
          }
          n438 = Unbundle By Name(w1014) -> ("code"=w1019:i32)
          n439 = Bundle By Name(cluster=w1018, "Data"=w1004, "Error #"=w1019) -> (w1017:T2)
        }
        frame "SetCLoad" {
          n440 = Unbundle By Name(w1050) -> ("Data"=w1043:T1)
          n441 = call-poly "CoreLib.byte array 2 data.vi"("byteArray"=w1043) -> ("i16"=w1039:i16, "error out"=w1038:errorcluster)  [unwired: 16 in, 1 out]
          n442 = Equal To 0?(x=w1039) -> (x = 0?=w1040:bool)
          n443 = Select(t=FALSE, s=w1040, f=TRUE) -> (s? t:f=w1037:bool)
          n444 = case shown="No Error" w1038 {
            tunnel: [w1059 w1067] -> w1048
            tunnel: w1053 -> [w1062 w1067]
            tunnel: w1052 -> [w1060 w1066]
            tunnel: [w1061 w1065] -> w1047
            tunnel: w1045 -> [_ w1064]
            tunnel: w1037 -> [w1063 _]
            frame No Error {
              n445 = call "DG535.set C load.vi"("i ref in"=w1062, "load"=w1063, "error in (no error)"=w1060) -> ("i ref out"=w1059:refnum<vi>, "error out"=w1061:errorcluster)  [unwired: 11 in]
            }
            frame Error {
              n446 = call "CoreLib.set data type mismatch.vi"("error in (no error)"=w1066, "error source"=w1064) -> ("error out"=w1065:errorcluster)  [unwired: 17 in]
            }
          }
          n447 = call "BaseProcess.set event status.vi"("i ref in"=w1048, "EventStatus"=w1045, "error in (no error)"=w1047) -> ("i ref out"=w1044:refnum<vi>, "error out"=w1046:errorcluster)  [unwired: 14 in, 1 out]
          n448 = case shown="Error" w1046 {
            selector: w1046 -> [_ w1058]
            tunnel: [w1054 w1056] -> w1036
            frame No Error {
              n449 = call-poly "CoreLib.data 2 byte array.vi"("string"="" ("source")) -> ("byteArray out"=w1054:T1)  [unwired: 18 in]
            }
            frame Error {
              n450 = Unbundle By Name(w1058) -> ("source"=w1057:string)
              n451 = call-poly "CoreLib.data 2 byte array.vi"("string"=w1057) -> ("byteArray out"=w1056:T1)  [unwired: 18 in]
            }
          }
          n452 = Unbundle By Name(w1046) -> ("code"=w1051:i32)
          n453 = Bundle By Name(cluster=w1050, "Data"=w1036, "Error #"=w1051) -> (w1049:T2)
        }
        frame "SetDLoad" {
          n454 = Unbundle By Name(w1082) -> ("Data"=w1075:T1)
          n455 = call-poly "CoreLib.byte array 2 data.vi"("byteArray"=w1075) -> ("i16"=w1071:i16, "error out"=w1070:errorcluster)  [unwired: 16 in, 1 out]
          n456 = Equal To 0?(x=w1071) -> (x = 0?=w1072:bool)
          n457 = Select(t=FALSE, s=w1072, f=TRUE) -> (s? t:f=w1069:bool)
          n458 = case shown="No Error" w1070 {
            tunnel: [w1091 w1099] -> w1080
            tunnel: w1085 -> [w1094 w1099]
            tunnel: w1084 -> [w1092 w1098]
            tunnel: [w1093 w1097] -> w1079
            tunnel: w1077 -> [_ w1096]
            tunnel: w1069 -> [w1095 _]
            frame No Error {
              n459 = call "DG535.set D load.vi"("i ref in"=w1094, "load"=w1095, "error in (no error)"=w1092) -> ("i ref out"=w1091:refnum<vi>, "error out"=w1093:errorcluster)  [unwired: 11 in]
            }
            frame Error {
              n460 = call "CoreLib.set data type mismatch.vi"("error in (no error)"=w1098, "error source"=w1096) -> ("error out"=w1097:errorcluster)  [unwired: 17 in]
            }
          }
          n461 = call "BaseProcess.set event status.vi"("i ref in"=w1080, "EventStatus"=w1077, "error in (no error)"=w1079) -> ("i ref out"=w1076:refnum<vi>, "error out"=w1078:errorcluster)  [unwired: 14 in, 1 out]
          n462 = case shown="Error" w1078 {
            selector: w1078 -> [_ w1090]
            tunnel: [w1086 w1088] -> w1068
            frame No Error {
              n463 = call-poly "CoreLib.data 2 byte array.vi"("string"="" ("source")) -> ("byteArray out"=w1086:T1)  [unwired: 18 in]
            }
            frame Error {
              n464 = Unbundle By Name(w1090) -> ("source"=w1089:string)
              n465 = call-poly "CoreLib.data 2 byte array.vi"("string"=w1089) -> ("byteArray out"=w1088:T1)  [unwired: 18 in]
            }
          }
          n466 = Unbundle By Name(w1078) -> ("code"=w1083:i32)
          n467 = Bundle By Name(cluster=w1082, "Data"=w1068, "Error #"=w1083) -> (w1081:T2)
        }
        frame "SetCDLoad" {
          n468 = Unbundle By Name(w1114) -> ("Data"=w1107:T1)
          n469 = call-poly "CoreLib.byte array 2 data.vi"("byteArray"=w1107) -> ("i16"=w1103:i16, "error out"=w1102:errorcluster)  [unwired: 16 in, 1 out]
          n470 = Equal To 0?(x=w1103) -> (x = 0?=w1104:bool)
          n471 = Select(t=FALSE, s=w1104, f=TRUE) -> (s? t:f=w1101:bool)
          n472 = case shown="No Error" w1102 {
            tunnel: [w1123 w1131] -> w1112
            tunnel: w1117 -> [w1126 w1131]
            tunnel: w1116 -> [w1124 w1130]
            tunnel: [w1125 w1129] -> w1111
            tunnel: w1109 -> [_ w1128]
            tunnel: w1101 -> [w1127 _]
            frame No Error {
              n473 = call "DG535.set CD load.vi"("i ref in"=w1126, "load"=w1127, "error in (no error)"=w1124) -> ("i ref out"=w1123:refnum<vi>, "error out"=w1125:errorcluster)  [unwired: 11 in]
            }
            frame Error {
              n474 = call "CoreLib.set data type mismatch.vi"("error in (no error)"=w1130, "error source"=w1128) -> ("error out"=w1129:errorcluster)  [unwired: 17 in]
            }
          }
          n475 = call "BaseProcess.set event status.vi"("i ref in"=w1112, "EventStatus"=w1109, "error in (no error)"=w1111) -> ("i ref out"=w1108:refnum<vi>, "error out"=w1110:errorcluster)  [unwired: 14 in, 1 out]
          n476 = case shown="No Error" w1110 {
            selector: w1110 -> [_ w1122]
            tunnel: [w1118 w1121] -> w1100
            frame No Error {
              n477 = call-poly "CoreLib.data 2 byte array.vi"("string"="" ("source")) -> ("byteArray out"=w1118:T1)  [unwired: 18 in]
            }
            frame Error {
              n478 = Unbundle By Name(w1122) -> ("source"=w1120:string)
              n479 = call-poly "CoreLib.data 2 byte array.vi"("string"=w1120) -> ("byteArray out"=w1121:T1)  [unwired: 18 in]
            }
          }
          n480 = Unbundle By Name(w1110) -> ("code"=w1115:i32)
          n481 = Bundle By Name(cluster=w1114, "Data"=w1100, "Error #"=w1115) -> (w1113:T2)
        }
        frame "SetDelay" {
          n482 = Unbundle By Name(w1141) -> ("Data"=w1132:T1)
          n483 = call-poly "CoreLib.byte array 2 data.vi"("byteArray"=w1132) -> ("d64"=w1140:dbl, "error out"=w1134:errorcluster)  [unwired: 16 in, 1 out]
          n484 = case shown="No Error" w1134 {
            tunnel: w1144 -> [w1147 w1154]
            tunnel: w1143 -> [w1149 w1153]
            tunnel: w1140 -> [w1148 _]
            tunnel: [w1146 w1154] -> w1139
            tunnel: [w1150 w1152] -> w1137
            tunnel: w1133 -> [_ w1151]
            frame No Error {
              n485 = call "DG535.SetDelay.vi"("i ref in"=w1147, "A Delay"=w1148, "error in (no error)"=w1149) -> ("i ref out"=w1146:refnum<vi>, "error out"=w1150:errorcluster)  [unwired: 11 in]
            }
            frame Error {
              n486 = call "CoreLib.set data type mismatch.vi"("error in (no error)"=w1153, "error source"=w1151) -> ("error out"=w1152:errorcluster)  [unwired: 17 in]
            }
          }
          n487 = call "BaseProcess.set event status.vi"("i ref in"=w1139, "EventStatus"=w1133, "error in (no error)"=w1137) -> ("i ref out"=w1138:refnum<vi>, "error out"=w1136:errorcluster)  [unwired: 14 in, 1 out]
          n488 = case shown="No Error" w1136 {
            selector: w1136 -> [_ w1159]
            tunnel: [w1155 w1157] -> w1142
            frame No Error {
              n489 = call-poly "CoreLib.data 2 byte array.vi"("string"="" ("source")) -> ("byteArray out"=w1155:T1)  [unwired: 18 in]
            }
            frame Error {
              n490 = Unbundle By Name(w1159) -> ("source"=w1158:string)
              n491 = call-poly "CoreLib.data 2 byte array.vi"("string"=w1158) -> ("byteArray out"=w1157:T1)  [unwired: 18 in]
            }
          }
          n492 = Unbundle By Name(w1136) -> ("code"=w1145:i32)
          n493 = Bundle By Name(cluster=w1141, "Data"=w1142, "Error #"=w1145) -> (w1135:T2)
        }
        frame "SetADelay" {
          n494 = Unbundle By Name(w1173) -> ("Data"=w1166:T1)
          n495 = call-poly "CoreLib.byte array 2 data.vi"("byteArray"=w1166) -> ("byteArray out"=w1163:T1, "string"=w1162:string, "error out"=w1165:errorcluster)  [unwired: 16 in]
          n496 = call-poly "CoreLib.byte array 2 data.vi"("byteArray"=w1163, "error in (no error)"=w1165) -> ("d64"=w1161:dbl, "error out"=w1164:errorcluster)  [unwired: 15 in, 1 out]
          n497 = case shown="Error" w1164 {
            tunnel: [w1186 w1191] -> w1171
            tunnel: w1176 -> [w1187 w1191]
            tunnel: w1175 -> [w1184 w1190]
            tunnel: [w1185 w1189] -> w1170
            tunnel: w1161 -> [w1182 _]
            tunnel: w1168 -> [_ w1188]
            tunnel: w1162 -> [w1183 _]
            frame No Error {
              n498 = call "DG535.set A delay.vi"("i ref in"=w1187, "Ref Channel"=w1183, "A Delay"=w1182, "error in (no error)"=w1184) -> ("i ref out"=w1186:refnum<vi>, "error out"=w1185:errorcluster)  [unwired: 10 in]
            }
            frame Error {
              n499 = call "CoreLib.set data type mismatch.vi"("error in (no error)"=w1190, "error source"=w1188) -> ("error out"=w1189:errorcluster)  [unwired: 17 in]
            }
          }
          n500 = call "BaseProcess.set event status.vi"("i ref in"=w1171, "EventStatus"=w1168, "error in (no error)"=w1170) -> ("i ref out"=w1167:refnum<vi>, "error out"=w1169:errorcluster)  [unwired: 14 in, 1 out]
          n501 = case shown="No Error" w1169 {
            selector: w1169 -> [_ w1181]
            tunnel: [w1177 w1179] -> w1160
            frame No Error {
              n502 = call-poly "CoreLib.data 2 byte array.vi"("string"="" ("source")) -> ("byteArray out"=w1177:T1)  [unwired: 18 in]
            }
            frame Error {
              n503 = Unbundle By Name(w1181) -> ("source"=w1180:string)
              n504 = call-poly "CoreLib.data 2 byte array.vi"("string"=w1180) -> ("byteArray out"=w1179:T1)  [unwired: 18 in]
            }
          }
          n505 = Unbundle By Name(w1169) -> ("code"=w1174:i32)
          n506 = Bundle By Name(cluster=w1173, "Data"=w1160, "Error #"=w1174) -> (w1172:T2)
        }
        frame "SetBDelay" {
          n507 = Unbundle By Name(w1205) -> ("Data"=w1198:T1)
          n508 = call-poly "CoreLib.byte array 2 data.vi"("byteArray"=w1198) -> ("byteArray out"=w1196:T1, "string"=w1195:string, "error out"=w1197:errorcluster)  [unwired: 16 in]
          n509 = call-poly "CoreLib.byte array 2 data.vi"("byteArray"=w1196, "error in (no error)"=w1197) -> ("d64"=w1194:dbl, "error out"=w1193:errorcluster)  [unwired: 15 in, 1 out]
          n510 = case shown="No Error" w1193 {
            tunnel: [w1218 w1223] -> w1203
            tunnel: w1208 -> [w1219 w1223]
            tunnel: w1207 -> [w1216 w1222]
            tunnel: [w1217 w1221] -> w1202
            tunnel: w1200 -> [_ w1220]
            tunnel: w1195 -> [w1215 _]
            tunnel: w1194 -> [w1214 _]
            frame No Error {
              n511 = call "DG535.set B delay.vi"("i ref in"=w1219, "Ref Channel"=w1215, "B Delay"=w1214, "error in (no error)"=w1216) -> ("i ref out"=w1218:refnum<vi>, "error out"=w1217:errorcluster)  [unwired: 10 in]
            }
            frame Error {
              n512 = call "CoreLib.set data type mismatch.vi"("error in (no error)"=w1222, "error source"=w1220) -> ("error out"=w1221:errorcluster)  [unwired: 17 in]
            }
          }
          n513 = call "BaseProcess.set event status.vi"("i ref in"=w1203, "EventStatus"=w1200, "error in (no error)"=w1202) -> ("i ref out"=w1199:refnum<vi>, "error out"=w1201:errorcluster)  [unwired: 14 in, 1 out]
          n514 = case shown="Error" w1201 {
            selector: w1201 -> [_ w1213]
            tunnel: [w1209 w1211] -> w1192
            frame No Error {
              n515 = call-poly "CoreLib.data 2 byte array.vi"("string"="" ("source")) -> ("byteArray out"=w1209:T1)  [unwired: 18 in]
            }
            frame Error {
              n516 = Unbundle By Name(w1213) -> ("source"=w1212:string)
              n517 = call-poly "CoreLib.data 2 byte array.vi"("string"=w1212) -> ("byteArray out"=w1211:T1)  [unwired: 18 in]
            }
          }
          n518 = Unbundle By Name(w1201) -> ("code"=w1206:i32)
          n519 = Bundle By Name(cluster=w1205, "Data"=w1192, "Error #"=w1206) -> (w1204:T2)
        }
        frame "SetCDelay" {
          n520 = Unbundle By Name(w1237) -> ("Data"=w1230:T1)
          n521 = call-poly "CoreLib.byte array 2 data.vi"("byteArray"=w1230) -> ("byteArray out"=w1228:T1, "string"=w1225:string, "error out"=w1229:errorcluster)  [unwired: 16 in]
          n522 = call-poly "CoreLib.byte array 2 data.vi"("byteArray"=w1228, "error in (no error)"=w1229) -> ("d64"=w1226:dbl, "error out"=w1227:errorcluster)  [unwired: 15 in, 1 out]
          n523 = case shown="No Error" w1227 {
            tunnel: [w1250 w1255] -> w1235
            tunnel: w1240 -> [w1251 w1255]
            tunnel: w1239 -> [w1248 w1254]
            tunnel: [w1249 w1253] -> w1234
            tunnel: w1226 -> [w1246 _]
            tunnel: w1232 -> [_ w1252]
            tunnel: w1225 -> [w1247 _]
            frame No Error {
              n524 = call "DG535.set C delay.vi"("i ref in"=w1251, "Ref Channel"=w1247, "C Delay"=w1246, "error in (no error)"=w1248) -> ("i ref out"=w1250:refnum<vi>, "error out"=w1249:errorcluster)  [unwired: 10 in]
            }
            frame Error {
              n525 = call "CoreLib.set data type mismatch.vi"("error in (no error)"=w1254, "error source"=w1252) -> ("error out"=w1253:errorcluster)  [unwired: 17 in]
            }
          }
          n526 = call "BaseProcess.set event status.vi"("i ref in"=w1235, "EventStatus"=w1232, "error in (no error)"=w1234) -> ("i ref out"=w1231:refnum<vi>, "error out"=w1233:errorcluster)  [unwired: 14 in, 1 out]
          n527 = case shown="Error" w1233 {
            selector: w1233 -> [_ w1245]
            tunnel: [w1241 w1243] -> w1224
            frame No Error {
              n528 = call-poly "CoreLib.data 2 byte array.vi"("string"="" ("source")) -> ("byteArray out"=w1241:T1)  [unwired: 18 in]
            }
            frame Error {
              n529 = Unbundle By Name(w1245) -> ("source"=w1244:string)
              n530 = call-poly "CoreLib.data 2 byte array.vi"("string"=w1244) -> ("byteArray out"=w1243:T1)  [unwired: 18 in]
            }
          }
          n531 = Unbundle By Name(w1233) -> ("code"=w1238:i32)
          n532 = Bundle By Name(cluster=w1237, "Data"=w1224, "Error #"=w1238) -> (w1236:T2)
        }
        frame "SetDDelay" {
          n533 = Unbundle By Name(w1269) -> ("Data"=w1262:T1)
          n534 = call-poly "CoreLib.byte array 2 data.vi"("byteArray"=w1262) -> ("byteArray out"=w1261:T1, "string"=w1259:string, "error out"=w1260:errorcluster)  [unwired: 16 in]
          n535 = call-poly "CoreLib.byte array 2 data.vi"("byteArray"=w1261, "error in (no error)"=w1260) -> ("d64"=w1257:dbl, "error out"=w1258:errorcluster)  [unwired: 15 in, 1 out]
          n536 = case shown="No Error" w1258 {
            tunnel: [w1282 w1287] -> w1267
            tunnel: w1272 -> [w1283 w1287]
            tunnel: w1271 -> [w1280 w1286]
            tunnel: [w1281 w1285] -> w1266
            tunnel: w1257 -> [w1278 _]
            tunnel: w1264 -> [_ w1284]
            tunnel: w1259 -> [w1279 _]
            frame No Error {
              n537 = call "DG535.set D delay.vi"("i ref in"=w1283, "Ref Channel"=w1279, "D Delay"=w1278, "error in (no error)"=w1280) -> ("i ref out"=w1282:refnum<vi>, "error out"=w1281:errorcluster)  [unwired: 10 in]
            }
            frame Error {
              n538 = call "CoreLib.set data type mismatch.vi"("error in (no error)"=w1286, "error source"=w1284) -> ("error out"=w1285:errorcluster)  [unwired: 17 in]
            }
          }
          n539 = call "BaseProcess.set event status.vi"("i ref in"=w1267, "EventStatus"=w1264, "error in (no error)"=w1266) -> ("i ref out"=w1263:refnum<vi>, "error out"=w1265:errorcluster)  [unwired: 14 in, 1 out]
          n540 = case shown="Error" w1265 {
            selector: w1265 -> [_ w1277]
            tunnel: [w1273 w1275] -> w1256
            frame No Error {
              n541 = call-poly "CoreLib.data 2 byte array.vi"("string"="" ("source")) -> ("byteArray out"=w1273:T1)  [unwired: 18 in]
            }
            frame Error {
              n542 = Unbundle By Name(w1277) -> ("source"=w1276:string)
              n543 = call-poly "CoreLib.data 2 byte array.vi"("string"=w1276) -> ("byteArray out"=w1275:T1)  [unwired: 18 in]
            }
          }
          n544 = Unbundle By Name(w1265) -> ("code"=w1270:i32)
          n545 = Bundle By Name(cluster=w1269, "Data"=w1256, "Error #"=w1270) -> (w1268:T2)
        }
        frame "GetT0Load" {
          n546 = call "DG535.get T0 load.vi"("i ref in"=w1293, "error in (no error)"=w1294) -> ("i ref out"=w1292:refnum<vi>, "load"=w1290:bool, "error out"=w1291:errorcluster)  [unwired: 11 in]
          n547 = call "BaseProcess.set event status.vi"("i ref in"=w1292, "EventStatus"=w1296, "error in (no error)"=w1291) -> ("i ref out"=w1295:refnum<vi>, "error out"=w1297:errorcluster)  [unwired: 14 in, 1 out]
          n548 = case shown="Error" w1297 {
            selector: w1297 -> [_ w1306]
            tunnel: [w1301 w1304] -> w1289
            tunnel: w1290 -> [w1303 _]
            frame No Error {
              n549 = Boolean To (0,1)(Boolean=w1303) -> (0, 1=w1302:i16)
              n550 = call-poly "CoreLib.data 2 byte array.vi"("i16"=w1302) -> ("byteArray out"=w1301:T1)  [unwired: 18 in]
            }
            frame Error {
              n551 = Unbundle By Name(w1306) -> ("source"=w1305:string)
              n552 = call-poly "CoreLib.data 2 byte array.vi"("string"=w1305) -> ("byteArray out"=w1304:T1)  [unwired: 18 in]
            }
          }
          n553 = Unbundle By Name(w1297) -> ("code"=w1300:i32)
          n554 = Bundle By Name(cluster=w1299, "Data"=w1289, "Error #"=w1300, "Data Descriptor"=T3 "S:1") -> (w1298:T2)
        }
        frame "GetALoad" {
          n555 = call "DG535.get A load.vi"("i ref in"=w1312, "error in (no error)"=w1313) -> ("i ref out"=w1311:refnum<vi>, "load"=w1309:bool, "error out"=w1310:errorcluster)  [unwired: 11 in]
          n556 = call "BaseProcess.set event status.vi"("i ref in"=w1311, "EventStatus"=w1315, "error in (no error)"=w1310) -> ("i ref out"=w1314:refnum<vi>, "error out"=w1316:errorcluster)  [unwired: 14 in, 1 out]
          n557 = case shown="Error" w1316 {
            selector: w1316 -> [_ w1325]
            tunnel: [w1320 w1323] -> w1308
            tunnel: w1309 -> [w1321 _]
            frame No Error {
              n558 = Boolean To (0,1)(Boolean=w1321) -> (0, 1=w1322:i16)
              n559 = call-poly "CoreLib.data 2 byte array.vi"("i16"=w1322) -> ("byteArray out"=w1320:T1)  [unwired: 18 in]
            }
            frame Error {
              n560 = Unbundle By Name(w1325) -> ("source"=w1324:string)
              n561 = call-poly "CoreLib.data 2 byte array.vi"("string"=w1324) -> ("byteArray out"=w1323:T1)  [unwired: 18 in]
            }
          }
          n562 = Unbundle By Name(w1316) -> ("code"=w1319:i32)
          n563 = Bundle By Name(cluster=w1318, "Data"=w1308, "Error #"=w1319, "Data Descriptor"=T3 "S:1") -> (w1317:T2)
        }
        frame "GetBLoad" {
          n564 = call "DG535.get B load.vi"("i ref in"=w1331, "error in (no error)"=w1332) -> ("i ref out"=w1330:refnum<vi>, "load"=w1328:bool, "error out"=w1329:errorcluster)  [unwired: 11 in]
          n565 = call "BaseProcess.set event status.vi"("i ref in"=w1330, "EventStatus"=w1334, "error in (no error)"=w1329) -> ("i ref out"=w1333:refnum<vi>, "error out"=w1335:errorcluster)  [unwired: 14 in, 1 out]
          n566 = case shown="No Error" w1335 {
            selector: w1335 -> [_ w1344]
            tunnel: [w1339 w1342] -> w1327
            tunnel: w1328 -> [w1341 _]
            frame No Error {
              n567 = Boolean To (0,1)(Boolean=w1341) -> (0, 1=w1340:i16)
              n568 = call-poly "CoreLib.data 2 byte array.vi"("i16"=w1340) -> ("byteArray out"=w1339:T1)  [unwired: 18 in]
            }
            frame Error {
              n569 = Unbundle By Name(w1344) -> ("source"=w1343:string)
              n570 = call-poly "CoreLib.data 2 byte array.vi"("string"=w1343) -> ("byteArray out"=w1342:T1)  [unwired: 18 in]
            }
          }
          n571 = Unbundle By Name(w1335) -> ("code"=w1338:i32)
          n572 = Bundle By Name(cluster=w1337, "Data"=w1327, "Error #"=w1338, "Data Descriptor"=T3 "S:1") -> (w1336:T2)
        }
        frame "GetABLoad" {
          n573 = call "DG535.get AB load.vi"("i ref in"=w1350, "error in (no error)"=w1351) -> ("i ref out"=w1349:refnum<vi>, "load"=w1347:bool, "error out"=w1348:errorcluster)  [unwired: 11 in]
          n574 = call "BaseProcess.set event status.vi"("i ref in"=w1349, "EventStatus"=w1353, "error in (no error)"=w1348) -> ("i ref out"=w1352:refnum<vi>, "error out"=w1354:errorcluster)  [unwired: 14 in, 1 out]
          n575 = case shown="No Error" w1354 {
            selector: w1354 -> [_ w1363]
            tunnel: [w1358 w1361] -> w1346
            tunnel: w1347 -> [w1360 _]
            frame No Error {
              n576 = Boolean To (0,1)(Boolean=w1360) -> (0, 1=w1359:i16)
              n577 = call-poly "CoreLib.data 2 byte array.vi"("i16"=w1359) -> ("byteArray out"=w1358:T1)  [unwired: 18 in]
            }
            frame Error {
              n578 = Unbundle By Name(w1363) -> ("source"=w1362:string)
              n579 = call-poly "CoreLib.data 2 byte array.vi"("string"=w1362) -> ("byteArray out"=w1361:T1)  [unwired: 18 in]
            }
          }
          n580 = Unbundle By Name(w1354) -> ("code"=w1357:i32)
          n581 = Bundle By Name(cluster=w1356, "Data"=w1346, "Error #"=w1357, "Data Descriptor"=T3 "S:1") -> (w1355:T2)
        }
        frame "GetCLoad" {
          n582 = call "DG535.get C load.vi"("i ref in"=w1369, "error in (no error)"=w1370) -> ("i ref out"=w1368:refnum<vi>, "load"=w1366:bool, "error out"=w1367:errorcluster)  [unwired: 11 in]
          n583 = call "BaseProcess.set event status.vi"("i ref in"=w1368, "EventStatus"=w1372, "error in (no error)"=w1367) -> ("i ref out"=w1371:refnum<vi>, "error out"=w1373:errorcluster)  [unwired: 14 in, 1 out]
          n584 = case shown="No Error" w1373 {
            selector: w1373 -> [_ w1382]
            tunnel: [w1377 w1380] -> w1365
            tunnel: w1366 -> [w1379 _]
            frame No Error {
              n585 = Boolean To (0,1)(Boolean=w1379) -> (0, 1=w1378:i16)
              n586 = call-poly "CoreLib.data 2 byte array.vi"("i16"=w1378) -> ("byteArray out"=w1377:T1)  [unwired: 18 in]
            }
            frame Error {
              n587 = Unbundle By Name(w1382) -> ("source"=w1381:string)
              n588 = call-poly "CoreLib.data 2 byte array.vi"("string"=w1381) -> ("byteArray out"=w1380:T1)  [unwired: 18 in]
            }
          }
          n589 = Unbundle By Name(w1373) -> ("code"=w1376:i32)
          n590 = Bundle By Name(cluster=w1375, "Data"=w1365, "Error #"=w1376, "Data Descriptor"=T3 "S:1") -> (w1374:T2)
        }
        frame "GetDLoad" {
          n591 = call "DG535.get D load.vi"("i ref in"=w1388, "error in (no error)"=w1389) -> ("i ref out"=w1387:refnum<vi>, "load"=w1385:bool, "error out"=w1386:errorcluster)  [unwired: 11 in]
          n592 = call "BaseProcess.set event status.vi"("i ref in"=w1387, "EventStatus"=w1391, "error in (no error)"=w1386) -> ("i ref out"=w1390:refnum<vi>, "error out"=w1392:errorcluster)  [unwired: 14 in, 1 out]
          n593 = case shown="Error" w1392 {
            selector: w1392 -> [_ w1401]
            tunnel: [w1396 w1400] -> w1384
            tunnel: w1385 -> [w1398 _]
            frame No Error {
              n594 = Boolean To (0,1)(Boolean=w1398) -> (0, 1=w1397:i16)
              n595 = call-poly "CoreLib.data 2 byte array.vi"("i16"=w1397) -> ("byteArray out"=w1396:T1)  [unwired: 18 in]
            }
            frame Error {
              n596 = Unbundle By Name(w1401) -> ("source"=w1399:string)
              n597 = call-poly "CoreLib.data 2 byte array.vi"("string"=w1399) -> ("byteArray out"=w1400:T1)  [unwired: 18 in]
            }
          }
          n598 = Unbundle By Name(w1392) -> ("code"=w1395:i32)
          n599 = Bundle By Name(cluster=w1394, "Data"=w1384, "Error #"=w1395, "Data Descriptor"=T3 "S:1") -> (w1393:T2)
        }
        frame "GetCDLoad" {
          n600 = call "DG535.get CD load.vi"("i ref in"=w1407, "error in (no error)"=w1408) -> ("i ref out"=w1406:refnum<vi>, "load"=w1404:bool, "error out"=w1405:errorcluster)  [unwired: 11 in]
          n601 = call "BaseProcess.set event status.vi"("i ref in"=w1406, "EventStatus"=w1410, "error in (no error)"=w1405) -> ("i ref out"=w1409:refnum<vi>, "error out"=w1411:errorcluster)  [unwired: 14 in, 1 out]
          n602 = case shown="No Error" w1411 {
            selector: w1411 -> [_ w1420]
            tunnel: [w1415 w1418] -> w1402
            tunnel: w1404 -> [w1417 _]
            frame No Error {
              n603 = Boolean To (0,1)(Boolean=w1417) -> (0, 1=w1416:i16)
              n604 = call-poly "CoreLib.data 2 byte array.vi"("i16"=w1416) -> ("byteArray out"=w1415:T1)  [unwired: 18 in]
            }
            frame Error {
              n605 = Unbundle By Name(w1420) -> ("source"=w1419:string)
              n606 = call-poly "CoreLib.data 2 byte array.vi"("string"=w1419) -> ("byteArray out"=w1418:T1)  [unwired: 18 in]
            }
          }
          n607 = Unbundle By Name(w1411) -> ("code"=w1414:i32)
          n608 = Bundle By Name(cluster=w1413, "Data"=w1402, "Error #"=w1414, "Data Descriptor"=T3 "S:1") -> (w1412:T2)
        }
        frame "GetABPolarity" {
          n609 = call "DG535.get AB polarity.vi"("i ref in"=w1426, "error in (no error)"=w1427) -> ("i ref out"=w1425:refnum<vi>, "inversion"=w1423:bool, "error out"=w1424:errorcluster)  [unwired: 11 in]
          n610 = call "BaseProcess.set event status.vi"("i ref in"=w1425, "EventStatus"=w1429, "error in (no error)"=w1424) -> ("i ref out"=w1428:refnum<vi>, "error out"=w1430:errorcluster)  [unwired: 14 in, 1 out]
          n611 = case shown="No Error" w1430 {
            selector: w1430 -> [_ w1439]
            tunnel: [w1434 w1437] -> w1421
            tunnel: w1423 -> [w1436 _]
            frame No Error {
              n612 = Boolean To (0,1)(Boolean=w1436) -> (0, 1=w1435:i16)
              n613 = call-poly "CoreLib.data 2 byte array.vi"("i16"=w1435) -> ("byteArray out"=w1434:T1)  [unwired: 18 in]
            }
            frame Error {
              n614 = Unbundle By Name(w1439) -> ("source"=w1438:string)
              n615 = call-poly "CoreLib.data 2 byte array.vi"("string"=w1438) -> ("byteArray out"=w1437:T1)  [unwired: 18 in]
            }
          }
          n616 = Unbundle By Name(w1430) -> ("code"=w1433:i32)
          n617 = Bundle By Name(cluster=w1432, "Data"=w1421, "Error #"=w1433, "Data Descriptor"=T3 "S:1") -> (w1431:T2)
        }
        frame "GetCDPolarity" {
          n618 = call "DG535.get CD polarity.vi"("i ref in"=w1445, "error in (no error)"=w1446) -> ("i ref out"=w1444:refnum<vi>, "inversion"=w1442:bool, "error out"=w1443:errorcluster)  [unwired: 11 in]
          n619 = call "BaseProcess.set event status.vi"("i ref in"=w1444, "EventStatus"=w1448, "error in (no error)"=w1443) -> ("i ref out"=w1447:refnum<vi>, "error out"=w1449:errorcluster)  [unwired: 14 in, 1 out]
          n620 = case shown="Error" w1449 {
            selector: w1449 -> [_ w1458]
            tunnel: [w1453 w1456] -> w1441
            tunnel: w1442 -> [w1455 _]
            frame No Error {
              n621 = Boolean To (0,1)(Boolean=w1455) -> (0, 1=w1454:i16)
              n622 = call-poly "CoreLib.data 2 byte array.vi"("i16"=w1454) -> ("byteArray out"=w1453:T1)  [unwired: 18 in]
            }
            frame Error {
              n623 = Unbundle By Name(w1458) -> ("source"=w1457:string)
              n624 = call-poly "CoreLib.data 2 byte array.vi"("string"=w1457) -> ("byteArray out"=w1456:T1)  [unwired: 18 in]
            }
          }
          n625 = Unbundle By Name(w1449) -> ("code"=w1452:i32)
          n626 = Bundle By Name(cluster=w1451, "Data"=w1441, "Error #"=w1452, "Data Descriptor"=T3 "S:1") -> (w1450:T2)
        }
        frame "GetT0Amplitude" {
          n627 = call "DG535.get T0 amplitude.vi"("i ref in"=w1464, "error in (no error)"=w1465) -> ("i ref out"=w1463:refnum<vi>, "amplitude"=w1461:dbl, "error out"=w1462:errorcluster)  [unwired: 11 in]
          n628 = call "BaseProcess.set event status.vi"("i ref in"=w1463, "EventStatus"=w1467, "error in (no error)"=w1462) -> ("i ref out"=w1466:refnum<vi>, "error out"=w1468:errorcluster)  [unwired: 14 in, 1 out]
          n629 = case shown="No Error" w1468 {
            selector: w1468 -> [_ w1476]
            tunnel: [w1472 w1475] -> w1459
            tunnel: w1461 -> [w1473 _]
            frame No Error {
              n630 = call-poly "CoreLib.data 2 byte array.vi"("f64"=w1473) -> ("byteArray out"=w1472:T1)  [unwired: 18 in]
            }
            frame Error {
              n631 = Unbundle By Name(w1476) -> ("source"=w1474:string)
              n632 = call-poly "CoreLib.data 2 byte array.vi"("string"=w1474) -> ("byteArray out"=w1475:T1)  [unwired: 18 in]
            }
          }
          n633 = Unbundle By Name(w1468) -> ("code"=w1471:i32)
          n634 = Bundle By Name(cluster=w1470, "Data"=w1459, "Error #"=w1471, "Data Descriptor"=T3 "D:1") -> (w1469:T2)
        }
        frame "GetAAmplitude" {
          n635 = call "DG535.get A amplitude.vi"("i ref in"=w1482, "error in (no error)"=w1483) -> ("i ref out"=w1481:refnum<vi>, "amplitude"=w1479:dbl, "error out"=w1480:errorcluster)  [unwired: 11 in]
          n636 = call "BaseProcess.set event status.vi"("i ref in"=w1481, "EventStatus"=w1485, "error in (no error)"=w1480) -> ("i ref out"=w1484:refnum<vi>, "error out"=w1486:errorcluster)  [unwired: 14 in, 1 out]
          n637 = case shown="No Error" w1486 {
            selector: w1486 -> [_ w1494]
            tunnel: [w1490 w1492] -> w1477
            tunnel: w1479 -> [w1491 _]
            frame No Error {
              n638 = call-poly "CoreLib.data 2 byte array.vi"("f64"=w1491) -> ("byteArray out"=w1490:T1)  [unwired: 18 in]
            }
            frame Error {
              n639 = Unbundle By Name(w1494) -> ("source"=w1493:string)
              n640 = call-poly "CoreLib.data 2 byte array.vi"("string"=w1493) -> ("byteArray out"=w1492:T1)  [unwired: 18 in]
            }
          }
          n641 = Unbundle By Name(w1486) -> ("code"=w1489:i32)
          n642 = Bundle By Name(cluster=w1488, "Data"=w1477, "Error #"=w1489, "Data Descriptor"=T3 "D:1") -> (w1487:T2)
        }
        frame "GetBAmplitude" {
          n643 = call "DG535.get B amplitude.vi"("i ref in"=w1500, "error in (no error)"=w1501) -> ("i ref out"=w1499:refnum<vi>, "amplitude"=w1497:dbl, "error out"=w1498:errorcluster)  [unwired: 11 in]
          n644 = call "BaseProcess.set event status.vi"("i ref in"=w1499, "EventStatus"=w1503, "error in (no error)"=w1498) -> ("i ref out"=w1502:refnum<vi>, "error out"=w1504:errorcluster)  [unwired: 14 in, 1 out]
          n645 = case shown="No Error" w1504 {
            selector: w1504 -> [_ w1512]
            tunnel: [w1508 w1511] -> w1495
            tunnel: w1497 -> [w1509 _]
            frame No Error {
              n646 = call-poly "CoreLib.data 2 byte array.vi"("f64"=w1509) -> ("byteArray out"=w1508:T1)  [unwired: 18 in]
            }
            frame Error {
              n647 = Unbundle By Name(w1512) -> ("source"=w1510:string)
              n648 = call-poly "CoreLib.data 2 byte array.vi"("string"=w1510) -> ("byteArray out"=w1511:T1)  [unwired: 18 in]
            }
          }
          n649 = Unbundle By Name(w1504) -> ("code"=w1507:i32)
          n650 = Bundle By Name(cluster=w1506, "Data"=w1495, "Error #"=w1507, "Data Descriptor"=T3 "D:1") -> (w1505:T2)
        }
        frame "GetABAmplitude" {
          n651 = call "DG535.get AB amplitude.vi"("i ref in"=w1518, "error in (no error)"=w1519) -> ("i ref out"=w1517:refnum<vi>, "amplitude"=w1515:dbl, "error out"=w1516:errorcluster)  [unwired: 11 in]
          n652 = call "BaseProcess.set event status.vi"("i ref in"=w1517, "EventStatus"=w1521, "error in (no error)"=w1516) -> ("i ref out"=w1520:refnum<vi>, "error out"=w1522:errorcluster)  [unwired: 14 in, 1 out]
          n653 = case shown="No Error" w1522 {
            selector: w1522 -> [_ w1530]
            tunnel: [w1526 w1528] -> w1513
            tunnel: w1515 -> [w1527 _]
            frame No Error {
              n654 = call-poly "CoreLib.data 2 byte array.vi"("f64"=w1527) -> ("byteArray out"=w1526:T1)  [unwired: 18 in]
            }
            frame Error {
              n655 = Unbundle By Name(w1530) -> ("source"=w1529:string)
              n656 = call-poly "CoreLib.data 2 byte array.vi"("string"=w1529) -> ("byteArray out"=w1528:T1)  [unwired: 18 in]
            }
          }
          n657 = Unbundle By Name(w1522) -> ("code"=w1525:i32)
          n658 = Bundle By Name(cluster=w1524, "Data"=w1513, "Error #"=w1525, "Data Descriptor"=T3 "D:1") -> (w1523:T2)
        }
        frame "GetCAmplitude" {
          n659 = call "DG535.get C amplitude.vi"("i ref in"=w1536, "error in (no error)"=w1537) -> ("i ref out"=w1535:refnum<vi>, "amplitude"=w1533:dbl, "error out"=w1534:errorcluster)  [unwired: 11 in]
          n660 = call "BaseProcess.set event status.vi"("i ref in"=w1535, "EventStatus"=w1539, "error in (no error)"=w1534) -> ("i ref out"=w1538:refnum<vi>, "error out"=w1540:errorcluster)  [unwired: 14 in, 1 out]
          n661 = case shown="No Error" w1540 {
            selector: w1540 -> [_ w1548]
            tunnel: [w1544 w1546] -> w1532
            tunnel: w1533 -> [w1545 _]
            frame No Error {
              n662 = call-poly "CoreLib.data 2 byte array.vi"("f64"=w1545) -> ("byteArray out"=w1544:T1)  [unwired: 18 in]
            }
            frame Error {
              n663 = Unbundle By Name(w1548) -> ("source"=w1547:string)
              n664 = call-poly "CoreLib.data 2 byte array.vi"("string"=w1547) -> ("byteArray out"=w1546:T1)  [unwired: 18 in]
            }
          }
          n665 = Unbundle By Name(w1540) -> ("code"=w1543:i32)
          n666 = Bundle By Name(cluster=w1542, "Data"=w1532, "Error #"=w1543, "Data Descriptor"=T3 "D:1") -> (w1541:T2)
        }
        frame "GetDAmplitude" {
          n667 = call "DG535.get D amplitude.vi"("i ref in"=w1554, "error in (no error)"=w1555) -> ("i ref out"=w1553:refnum<vi>, "amplitude"=w1551:dbl, "error out"=w1552:errorcluster)  [unwired: 11 in]
          n668 = call "BaseProcess.set event status.vi"("i ref in"=w1553, "EventStatus"=w1557, "error in (no error)"=w1552) -> ("i ref out"=w1556:refnum<vi>, "error out"=w1558:errorcluster)  [unwired: 14 in, 1 out]
          n669 = case shown="No Error" w1558 {
            selector: w1558 -> [_ w1566]
            tunnel: [w1562 w1564] -> w1550
            tunnel: w1551 -> [w1563 _]
            frame No Error {
              n670 = call-poly "CoreLib.data 2 byte array.vi"("f64"=w1563) -> ("byteArray out"=w1562:T1)  [unwired: 18 in]
            }
            frame Error {
              n671 = Unbundle By Name(w1566) -> ("source"=w1565:string)
              n672 = call-poly "CoreLib.data 2 byte array.vi"("string"=w1565) -> ("byteArray out"=w1564:T1)  [unwired: 18 in]
            }
          }
          n673 = Unbundle By Name(w1558) -> ("code"=w1561:i32)
          n674 = Bundle By Name(cluster=w1560, "Data"=w1550, "Error #"=w1561, "Data Descriptor"=T3 "D:1") -> (w1559:T2)
        }
        frame "GetCDAmplitude" {
          n675 = call "DG535.get CD amplitude.vi"("i ref in"=w1572, "error in (no error)"=w1573) -> ("i ref out"=w1571:refnum<vi>, "amplitude"=w1569:dbl, "error out"=w1570:errorcluster)  [unwired: 11 in]
          n676 = call "BaseProcess.set event status.vi"("i ref in"=w1571, "EventStatus"=w1575, "error in (no error)"=w1570) -> ("i ref out"=w1574:refnum<vi>, "error out"=w1576:errorcluster)  [unwired: 14 in, 1 out]
          n677 = case shown="Error" w1576 {
            selector: w1576 -> [_ w1584]
            tunnel: [w1580 w1582] -> w1568
            tunnel: w1569 -> [w1581 _]
            frame No Error {
              n678 = call-poly "CoreLib.data 2 byte array.vi"("f64"=w1581) -> ("byteArray out"=w1580:T1)  [unwired: 18 in]
            }
            frame Error {
              n679 = Unbundle By Name(w1584) -> ("source"=w1583:string)
              n680 = call-poly "CoreLib.data 2 byte array.vi"("string"=w1583) -> ("byteArray out"=w1582:T1)  [unwired: 18 in]
            }
          }
          n681 = Unbundle By Name(w1576) -> ("code"=w1579:i32)
          n682 = Bundle By Name(cluster=w1578, "Data"=w1568, "Error #"=w1579, "Data Descriptor"=T3 "D:1") -> (w1577:T2)
        }
        frame "GetT0Offset" {
          n683 = call "DG535.get T0 offset.vi"("i ref in"=w1590, "error in (no error)"=w1591) -> ("i ref out"=w1589:refnum<vi>, "Offset"=w1587:dbl, "error out"=w1588:errorcluster)  [unwired: 11 in]
          n684 = call "BaseProcess.set event status.vi"("i ref in"=w1589, "EventStatus"=w1593, "error in (no error)"=w1588) -> ("i ref out"=w1592:refnum<vi>, "error out"=w1594:errorcluster)  [unwired: 14 in, 1 out]
          n685 = case shown="Error" w1594 {
            selector: w1594 -> [_ w1602]
            tunnel: [w1598 w1600] -> w1585
            tunnel: w1587 -> [w1599 _]
            frame No Error {
              n686 = call-poly "CoreLib.data 2 byte array.vi"("f64"=w1599) -> ("byteArray out"=w1598:T1)  [unwired: 18 in]
            }
            frame Error {
              n687 = Unbundle By Name(w1602) -> ("source"=w1601:string)
              n688 = call-poly "CoreLib.data 2 byte array.vi"("string"=w1601) -> ("byteArray out"=w1600:T1)  [unwired: 18 in]
            }
          }
          n689 = Unbundle By Name(w1594) -> ("code"=w1597:i32)
          n690 = Bundle By Name(cluster=w1596, "Data"=w1585, "Error #"=w1597, "Data Descriptor"=T3 "D:1") -> (w1595:T2)
        }
        frame "GetAOffset" {
          n691 = call "DG535.get A offset.vi"("i ref in"=w1608, "error in (no error)"=w1609) -> ("i ref out"=w1607:refnum<vi>, "Offset"=w1605:dbl, "error out"=w1606:errorcluster)  [unwired: 11 in]
          n692 = call "BaseProcess.set event status.vi"("i ref in"=w1607, "EventStatus"=w1611, "error in (no error)"=w1606) -> ("i ref out"=w1610:refnum<vi>, "error out"=w1612:errorcluster)  [unwired: 14 in, 1 out]
          n693 = case shown="No Error" w1612 {
            selector: w1612 -> [_ w1620]
            tunnel: [w1616 w1618] -> w1603
            tunnel: w1605 -> [w1617 _]
            frame No Error {
              n694 = call-poly "CoreLib.data 2 byte array.vi"("f64"=w1617) -> ("byteArray out"=w1616:T1)  [unwired: 18 in]
            }
            frame Error {
              n695 = Unbundle By Name(w1620) -> ("source"=w1619:string)
              n696 = call-poly "CoreLib.data 2 byte array.vi"("string"=w1619) -> ("byteArray out"=w1618:T1)  [unwired: 18 in]
            }
          }
          n697 = Unbundle By Name(w1612) -> ("code"=w1615:i32)
          n698 = Bundle By Name(cluster=w1614, "Data"=w1603, "Error #"=w1615, "Data Descriptor"=T3 "D:1") -> (w1613:T2)
        }
        frame "GetBOffset" {
          n699 = call "DG535.get B offset.vi"("i ref in"=w1626, "error in (no error)"=w1627) -> ("i ref out"=w1625:refnum<vi>, "Offset"=w1623:dbl, "error out"=w1624:errorcluster)  [unwired: 11 in]
          n700 = call "BaseProcess.set event status.vi"("i ref in"=w1625, "EventStatus"=w1629, "error in (no error)"=w1624) -> ("i ref out"=w1628:refnum<vi>, "error out"=w1630:errorcluster)  [unwired: 14 in, 1 out]
          n701 = case shown="No Error" w1630 {
            selector: w1630 -> [_ w1638]
            tunnel: [w1634 w1636] -> w1621
            tunnel: w1623 -> [w1635 _]
            frame No Error {
              n702 = call-poly "CoreLib.data 2 byte array.vi"("f64"=w1635) -> ("byteArray out"=w1634:T1)  [unwired: 18 in]
            }
            frame Error {
              n703 = Unbundle By Name(w1638) -> ("source"=w1637:string)
              n704 = call-poly "CoreLib.data 2 byte array.vi"("string"=w1637) -> ("byteArray out"=w1636:T1)  [unwired: 18 in]
            }
          }
          n705 = Unbundle By Name(w1630) -> ("code"=w1633:i32)
          n706 = Bundle By Name(cluster=w1632, "Data"=w1621, "Error #"=w1633, "Data Descriptor"=T3 "D:1") -> (w1631:T2)
        }
        frame "GetABOffset" {
          n707 = call "DG535.get AB offset.vi"("i ref in"=w1644, "error in (no error)"=w1645) -> ("i ref out"=w1643:refnum<vi>, "Offset"=w1641:dbl, "error out"=w1642:errorcluster)  [unwired: 11 in]
          n708 = call "BaseProcess.set event status.vi"("i ref in"=w1643, "EventStatus"=w1647, "error in (no error)"=w1642) -> ("i ref out"=w1646:refnum<vi>, "error out"=w1648:errorcluster)  [unwired: 14 in, 1 out]
          n709 = case shown="No Error" w1648 {
            selector: w1648 -> [_ w1656]
            tunnel: [w1652 w1654] -> w1639
            tunnel: w1641 -> [w1653 _]
            frame No Error {
              n710 = call-poly "CoreLib.data 2 byte array.vi"("f64"=w1653) -> ("byteArray out"=w1652:T1)  [unwired: 18 in]
            }
            frame Error {
              n711 = Unbundle By Name(w1656) -> ("source"=w1655:string)
              n712 = call-poly "CoreLib.data 2 byte array.vi"("string"=w1655) -> ("byteArray out"=w1654:T1)  [unwired: 18 in]
            }
          }
          n713 = Unbundle By Name(w1648) -> ("code"=w1651:i32)
          n714 = Bundle By Name(cluster=w1650, "Data"=w1639, "Error #"=w1651, "Data Descriptor"=T3 "D:1") -> (w1649:T2)
        }
        frame "GetCOffset" {
          n715 = call "DG535.get C offset.vi"("i ref in"=w1662, "error in (no error)"=w1663) -> ("i ref out"=w1661:refnum<vi>, "Offset"=w1659:dbl, "error out"=w1660:errorcluster)  [unwired: 11 in]
          n716 = call "BaseProcess.set event status.vi"("i ref in"=w1661, "EventStatus"=w1665, "error in (no error)"=w1660) -> ("i ref out"=w1664:refnum<vi>, "error out"=w1666:errorcluster)  [unwired: 14 in, 1 out]
          n717 = case shown="No Error" w1666 {
            selector: w1666 -> [_ w1674]
            tunnel: [w1670 w1672] -> w1657
            tunnel: w1659 -> [w1671 _]
            frame No Error {
              n718 = call-poly "CoreLib.data 2 byte array.vi"("f64"=w1671) -> ("byteArray out"=w1670:T1)  [unwired: 18 in]
            }
            frame Error {
              n719 = Unbundle By Name(w1674) -> ("source"=w1673:string)
              n720 = call-poly "CoreLib.data 2 byte array.vi"("string"=w1673) -> ("byteArray out"=w1672:T1)  [unwired: 18 in]
            }
          }
          n721 = Unbundle By Name(w1666) -> ("code"=w1669:i32)
          n722 = Bundle By Name(cluster=w1668, "Data"=w1657, "Error #"=w1669, "Data Descriptor"=T3 "D:1") -> (w1667:T2)
        }
        frame "GetDOffset" {
          n723 = call "DG535.get D offset.vi"("i ref in"=w1680, "error in (no error)"=w1681) -> ("i ref out"=w1679:refnum<vi>, "Offset"=w1677:dbl, "error out"=w1678:errorcluster)  [unwired: 11 in]
          n724 = call "BaseProcess.set event status.vi"("i ref in"=w1679, "EventStatus"=w1683, "error in (no error)"=w1678) -> ("i ref out"=w1682:refnum<vi>, "error out"=w1684:errorcluster)  [unwired: 14 in, 1 out]
          n725 = case shown="No Error" w1684 {
            selector: w1684 -> [_ w1692]
            tunnel: [w1688 w1691] -> w1675
            tunnel: w1677 -> [w1689 _]
            frame No Error {
              n726 = call-poly "CoreLib.data 2 byte array.vi"("f64"=w1689) -> ("byteArray out"=w1688:T1)  [unwired: 18 in]
            }
            frame Error {
              n727 = Unbundle By Name(w1692) -> ("source"=w1690:string)
              n728 = call-poly "CoreLib.data 2 byte array.vi"("string"=w1690) -> ("byteArray out"=w1691:T1)  [unwired: 18 in]
            }
          }
          n729 = Unbundle By Name(w1684) -> ("code"=w1687:i32)
          n730 = Bundle By Name(cluster=w1686, "Data"=w1675, "Error #"=w1687, "Data Descriptor"=T3 "D:1") -> (w1685:T2)
        }
        frame "GetCDOffset" {
          n731 = call "DG535.get CD offset.vi"("i ref in"=w1698, "error in (no error)"=w1699) -> ("i ref out"=w1697:refnum<vi>, "Offset"=w1695:dbl, "error out"=w1696:errorcluster)  [unwired: 11 in]
          n732 = call "BaseProcess.set event status.vi"("i ref in"=w1697, "EventStatus"=w1701, "error in (no error)"=w1696) -> ("i ref out"=w1700:refnum<vi>, "error out"=w1702:errorcluster)  [unwired: 14 in, 1 out]
          n733 = case shown="No Error" w1702 {
            selector: w1702 -> [_ w1710]
            tunnel: [w1706 w1709] -> w1693
            tunnel: w1695 -> [w1707 _]
            frame No Error {
              n734 = call-poly "CoreLib.data 2 byte array.vi"("f64"=w1707) -> ("byteArray out"=w1706:T1)  [unwired: 18 in]
            }
            frame Error {
              n735 = Unbundle By Name(w1710) -> ("source"=w1708:string)
              n736 = call-poly "CoreLib.data 2 byte array.vi"("string"=w1708) -> ("byteArray out"=w1709:T1)  [unwired: 18 in]
            }
          }
          n737 = Unbundle By Name(w1702) -> ("code"=w1705:i32)
          n738 = Bundle By Name(cluster=w1704, "Data"=w1693, "Error #"=w1705, "Data Descriptor"=T3 "D:1") -> (w1703:T2)
        }
        frame "GetT0Mode" {
          n739 = call "DG535.get T0 mode.vi"("i ref in"=w1716, "error in (no error)"=w1717) -> ("i ref out"=w1715:refnum<vi>, "mode"=w1713:i32, "error out"=w1714:errorcluster)  [unwired: 11 in]
          n740 = call "BaseProcess.set event status.vi"("i ref in"=w1715, "EventStatus"=w1719, "error in (no error)"=w1714) -> ("i ref out"=w1718:refnum<vi>, "error out"=w1720:errorcluster)  [unwired: 14 in, 1 out]
          n741 = case shown="No Error" w1720 {
            selector: w1720 -> [_ w1728]
            tunnel: [w1724 w1727] -> w1711
            tunnel: w1713 -> [w1725 _]
            frame No Error {
              n742 = call-poly "CoreLib.data 2 byte array.vi"("i32"=w1725) -> ("byteArray out"=w1724:T1)  [unwired: 18 in]
            }
            frame Error {
              n743 = Unbundle By Name(w1728) -> ("source"=w1726:string)
              n744 = call-poly "CoreLib.data 2 byte array.vi"("string"=w1726) -> ("byteArray out"=w1727:T1)  [unwired: 18 in]
            }
          }
          n745 = Unbundle By Name(w1720) -> ("code"=w1723:i32)
          n746 = Bundle By Name(cluster=w1722, "Data"=w1711, "Error #"=w1723, "Data Descriptor"=T3 "I:1") -> (w1721:T2)
        }
        frame "GetAMode" {
          n747 = call "DG535.get A mode.vi"("i ref in"=w1734, "error in (no error)"=w1735) -> ("i ref out"=w1733:refnum<vi>, "mode"=w1731:i32, "error out"=w1732:errorcluster)  [unwired: 11 in]
          n748 = call "BaseProcess.set event status.vi"("i ref in"=w1733, "EventStatus"=w1737, "error in (no error)"=w1732) -> ("i ref out"=w1736:refnum<vi>, "error out"=w1738:errorcluster)  [unwired: 14 in, 1 out]
          n749 = case shown="No Error" w1738 {
            selector: w1738 -> [_ w1746]
            tunnel: [w1742 w1744] -> w1730
            tunnel: w1731 -> [w1743 _]
            frame No Error {
              n750 = call-poly "CoreLib.data 2 byte array.vi"("i32"=w1743) -> ("byteArray out"=w1742:T1)  [unwired: 18 in]
            }
            frame Error {
              n751 = Unbundle By Name(w1746) -> ("source"=w1745:string)
              n752 = call-poly "CoreLib.data 2 byte array.vi"("string"=w1745) -> ("byteArray out"=w1744:T1)  [unwired: 18 in]
            }
          }
          n753 = Unbundle By Name(w1738) -> ("code"=w1741:i32)
          n754 = Bundle By Name(cluster=w1740, "Data"=w1730, "Error #"=w1741, "Data Descriptor"=T3 "I:1") -> (w1739:T2)
        }
        frame "GetBMode" {
          n755 = call "DG535.get B mode.vi"("i ref in"=w1752, "error in (no error)"=w1753) -> ("i ref out"=w1751:refnum<vi>, "mode"=w1749:i32, "error out"=w1750:errorcluster)  [unwired: 11 in]
          n756 = call "BaseProcess.set event status.vi"("i ref in"=w1751, "EventStatus"=w1755, "error in (no error)"=w1750) -> ("i ref out"=w1754:refnum<vi>, "error out"=w1756:errorcluster)  [unwired: 14 in, 1 out]
          n757 = case shown="No Error" w1756 {
            selector: w1756 -> [_ w1764]
            tunnel: [w1760 w1762] -> w1747
            tunnel: w1749 -> [w1761 _]
            frame No Error {
              n758 = call-poly "CoreLib.data 2 byte array.vi"("i32"=w1761) -> ("byteArray out"=w1760:T1)  [unwired: 18 in]
            }
            frame Error {
              n759 = Unbundle By Name(w1764) -> ("source"=w1763:string)
              n760 = call-poly "CoreLib.data 2 byte array.vi"("string"=w1763) -> ("byteArray out"=w1762:T1)  [unwired: 18 in]
            }
          }
          n761 = Unbundle By Name(w1756) -> ("code"=w1759:i32)
          n762 = Bundle By Name(cluster=w1758, "Data"=w1747, "Error #"=w1759, "Data Descriptor"=T3 "I:1") -> (w1757:T2)
        }
        frame "GetABMode" {
          n763 = call "DG535.get AB mode.vi"("i ref in"=w1770, "error in (no error)"=w1771) -> ("i ref out"=w1769:refnum<vi>, "mode"=w1767:i32, "error out"=w1768:errorcluster)  [unwired: 11 in]
          n764 = call "BaseProcess.set event status.vi"("i ref in"=w1769, "EventStatus"=w1773, "error in (no error)"=w1768) -> ("i ref out"=w1772:refnum<vi>, "error out"=w1774:errorcluster)  [unwired: 14 in, 1 out]
          n765 = case shown="Error" w1774 {
            selector: w1774 -> [_ w1782]
            tunnel: [w1778 w1780] -> w1766
            tunnel: w1767 -> [w1779 _]
            frame No Error {
              n766 = call-poly "CoreLib.data 2 byte array.vi"("i32"=w1779) -> ("byteArray out"=w1778:T1)  [unwired: 18 in]
            }
            frame Error {
              n767 = Unbundle By Name(w1782) -> ("source"=w1781:string)
              n768 = call-poly "CoreLib.data 2 byte array.vi"("string"=w1781) -> ("byteArray out"=w1780:T1)  [unwired: 18 in]
            }
          }
          n769 = Unbundle By Name(w1774) -> ("code"=w1777:i32)
          n770 = Bundle By Name(cluster=w1776, "Data"=w1766, "Error #"=w1777, "Data Descriptor"=T3 "I:1") -> (w1775:T2)
        }
        frame "GetCMode" {
          n771 = call "DG535.get C mode.vi"("i ref in"=w1788, "error in (no error)"=w1789) -> ("i ref out"=w1787:refnum<vi>, "mode"=w1785:i32, "error out"=w1786:errorcluster)  [unwired: 11 in]
          n772 = call "BaseProcess.set event status.vi"("i ref in"=w1787, "EventStatus"=w1791, "error in (no error)"=w1786) -> ("i ref out"=w1790:refnum<vi>, "error out"=w1792:errorcluster)  [unwired: 14 in, 1 out]
          n773 = case shown="Error" w1792 {
            selector: w1792 -> [_ w1800]
            tunnel: [w1796 w1798] -> w1784
            tunnel: w1785 -> [w1797 _]
            frame No Error {
              n774 = call-poly "CoreLib.data 2 byte array.vi"("i32"=w1797) -> ("byteArray out"=w1796:T1)  [unwired: 18 in]
            }
            frame Error {
              n775 = Unbundle By Name(w1800) -> ("source"=w1799:string)
              n776 = call-poly "CoreLib.data 2 byte array.vi"("string"=w1799) -> ("byteArray out"=w1798:T1)  [unwired: 18 in]
            }
          }
          n777 = Unbundle By Name(w1792) -> ("code"=w1795:i32)
          n778 = Bundle By Name(cluster=w1794, "Data"=w1784, "Error #"=w1795, "Data Descriptor"=T3 "I:1") -> (w1793:T2)
        }
        frame "GetDMode" {
          n779 = call "DG535.get D mode.vi"("i ref in"=w1806, "error in (no error)"=w1807) -> ("i ref out"=w1805:refnum<vi>, "mode"=w1803:i32, "error out"=w1804:errorcluster)  [unwired: 11 in]
          n780 = call "BaseProcess.set event status.vi"("i ref in"=w1805, "EventStatus"=w1809, "error in (no error)"=w1804) -> ("i ref out"=w1808:refnum<vi>, "error out"=w1810:errorcluster)  [unwired: 14 in, 1 out]
          n781 = case shown="Error" w1810 {
            selector: w1810 -> [_ w1818]
            tunnel: [w1814 w1817] -> w1801
            tunnel: w1803 -> [w1815 _]
            frame No Error {
              n782 = call-poly "CoreLib.data 2 byte array.vi"("i32"=w1815) -> ("byteArray out"=w1814:T1)  [unwired: 18 in]
            }
            frame Error {
              n783 = Unbundle By Name(w1818) -> ("source"=w1816:string)
              n784 = call-poly "CoreLib.data 2 byte array.vi"("string"=w1816) -> ("byteArray out"=w1817:T1)  [unwired: 18 in]
            }
          }
          n785 = Unbundle By Name(w1810) -> ("code"=w1813:i32)
          n786 = Bundle By Name(cluster=w1812, "Data"=w1801, "Error #"=w1813, "Data Descriptor"=T3 "I:1") -> (w1811:T2)
        }
        frame "GetCDMode" {
          n787 = call "DG535.get CD mode.vi"("i ref in"=w1824, "error in (no error)"=w1825) -> ("i ref out"=w1823:refnum<vi>, "mode"=w1821:i32, "error out"=w1822:errorcluster)  [unwired: 11 in]
          n788 = call "BaseProcess.set event status.vi"("i ref in"=w1823, "EventStatus"=w1827, "error in (no error)"=w1822) -> ("i ref out"=w1826:refnum<vi>, "error out"=w1828:errorcluster)  [unwired: 14 in, 1 out]
          n789 = case shown="No Error" w1828 {
            selector: w1828 -> [_ w1836]
            tunnel: [w1832 w1834] -> w1819
            tunnel: w1821 -> [w1833 _]
            frame No Error {
              n790 = call-poly "CoreLib.data 2 byte array.vi"("i32"=w1833) -> ("byteArray out"=w1832:T1)  [unwired: 18 in]
            }
            frame Error {
              n791 = Unbundle By Name(w1836) -> ("source"=w1835:string)
              n792 = call-poly "CoreLib.data 2 byte array.vi"("string"=w1835) -> ("byteArray out"=w1834:T1)  [unwired: 18 in]
            }
          }
          n793 = Unbundle By Name(w1828) -> ("code"=w1831:i32)
          n794 = Bundle By Name(cluster=w1830, "Data"=w1819, "Error #"=w1831, "Data Descriptor"=T3 "I:1") -> (w1829:T2)
        }
        frame "SetDelays" {
          n795 = Unbundle By Name(w1868) -> ("Data"=w1860:T1)
          n796 = call-poly "CoreLib.byte array 2 data.vi"("byteArray"=w1860) -> ("byteArray out"=w1858:T1, "i32"=w1859:i32, "error out"=w1857:errorcluster)  [unwired: 16 in]
          n797 = call-poly "CoreLib.byte array 2 data.vi"("byteArray"=w1858, "error in (no error)"=w1857) -> ("byteArray out"=w1855:T1, "d64"=w1856:dbl, "error out"=w1854:errorcluster)  [unwired: 15 in]
          n798 = call-poly "CoreLib.byte array 2 data.vi"("byteArray"=w1855, "error in (no error)"=w1854) -> ("byteArray out"=w1853:T1, "i32"=w1843:i32, "error out"=w1852:errorcluster)  [unwired: 15 in]
          n799 = call-poly "CoreLib.byte array 2 data.vi"("byteArray"=w1853, "error in (no error)"=w1852) -> ("byteArray out"=w1850:T1, "d64"=w1842:dbl, "error out"=w1851:errorcluster)  [unwired: 15 in]
          n800 = call-poly "CoreLib.byte array 2 data.vi"("byteArray"=w1850, "error in (no error)"=w1851) -> ("byteArray out"=w1848:T1, "i32"=w1841:i32, "error out"=w1849:errorcluster)  [unwired: 15 in]
          n801 = call-poly "CoreLib.byte array 2 data.vi"("byteArray"=w1848, "error in (no error)"=w1849) -> ("byteArray out"=w1846:T1, "d64"=w1840:dbl, "error out"=w1847:errorcluster)  [unwired: 15 in]
          n802 = call-poly "CoreLib.byte array 2 data.vi"("byteArray"=w1846, "error in (no error)"=w1847) -> ("byteArray out"=w1844:T1, "i32"=w1839:i32, "error out"=w1845:errorcluster)  [unwired: 15 in]
          n803 = call-poly "CoreLib.byte array 2 data.vi"("byteArray"=w1844, "error in (no error)"=w1845) -> ("d64"=w1838:dbl, "error out"=w1837:errorcluster)  [unwired: 15 in, 1 out]
          n804 = case shown="No Error" w1837 {
            tunnel: [w1887 w1892] -> w1866
            tunnel: w1871 -> [w1888 w1892]
            tunnel: w1870 -> [w1885 w1891]
            tunnel: [w1886 w1890] -> w1865
            tunnel: w1863 -> [_ w1889]
            tunnel: w1859 -> [w1880 _]
            tunnel: w1856 -> [w1879 _]
            tunnel: w1843 -> [w1878 _]
            tunnel: w1842 -> [w1877 _]
            tunnel: w1841 -> [w1884 _]
            tunnel: w1840 -> [w1883 _]
            tunnel: w1839 -> [w1881 _]
            tunnel: w1838 -> [w1882 _]
            frame No Error {
              # "D"
              # "C"
              # "B"
              # "A"
              n805 = call "DG535.set delays.vi"("i ref in"=w1888, "A="=w1880, "A"=w1879, "B="=w1878, "B"=w1877, "error in (no error)"=w1885, "D="=w1881, "C="=w1884, "D"=w1882, "C"=w1883) -> ("i ref out"=w1887:refnum<vi>, "error out"=w1886:errorcluster)  [unwired: 8 in]
            }
            frame Error {
              n806 = call "CoreLib.set data type mismatch.vi"("error in (no error)"=w1891, "error source"=w1889) -> ("error out"=w1890:errorcluster)  [unwired: 17 in]
            }
          }
          n807 = call "BaseProcess.set event status.vi"("i ref in"=w1866, "EventStatus"=w1863, "error in (no error)"=w1865) -> ("i ref out"=w1862:refnum<vi>, "error out"=w1864:errorcluster)  [unwired: 14 in, 1 out]
          n808 = case shown="Error" w1864 {
            selector: w1864 -> [_ w1876]
            tunnel: [w1872 w1874] -> w1861
            frame No Error {
              n809 = call-poly "CoreLib.data 2 byte array.vi"("string"="" ("source")) -> ("byteArray out"=w1872:T1)  [unwired: 18 in]
            }
            frame Error {
              n810 = Unbundle By Name(w1876) -> ("source"=w1875:string)
              n811 = call-poly "CoreLib.data 2 byte array.vi"("string"=w1875) -> ("byteArray out"=w1874:T1)  [unwired: 18 in]
            }
          }
          n812 = Unbundle By Name(w1864) -> ("code"=w1869:i32)
          n813 = Bundle By Name(cluster=w1868, "Data"=w1861, "Error #"=w1869) -> (w1867:T2)
        }
        frame "SetOutputs" {
          n814 = Unbundle By Name(w1933) -> ("Data"=w1911:T1)
          n815 = call-poly "CoreLib.byte array 2 data.vi"("byteArray"=w1911) -> ("byteArray out"=w1923:T1, "i16"=w1894:i16, "error out"=w1922:errorcluster)  [unwired: 16 in]
          n816 = call-poly "CoreLib.byte array 2 data.vi"("byteArray"=w1923, "error in (no error)"=w1922) -> ("byteArray out"=w1921:T1, "i32"=w1896:i32, "error out"=w1920:errorcluster)  [unwired: 15 in]
          n817 = call-poly "CoreLib.byte array 2 data.vi"("byteArray"=w1921, "error in (no error)"=w1920) -> ("byteArray out"=w1919:T1, "i32"=w1897:i32, "error out"=w1918:errorcluster)  [unwired: 15 in]
          n818 = call-poly "CoreLib.byte array 2 data.vi"("byteArray"=w1919, "error in (no error)"=w1918) -> ("byteArray out"=w1916:T1, "d64"=w1898:dbl, "error out"=w1917:errorcluster)  [unwired: 15 in]
          n819 = call-poly "CoreLib.byte array 2 data.vi"("byteArray"=w1916, "error in (no error)"=w1917) -> ("byteArray out"=w1914:T1, "d64"=w1899:dbl, "error out"=w1915:errorcluster)  [unwired: 15 in]
          n820 = call-poly "CoreLib.byte array 2 data.vi"("byteArray"=w1914, "error in (no error)"=w1915) -> ("byteArray out"=w1912:T1, "i16"=w1900:i16, "error out"=w1913:errorcluster)  [unwired: 15 in]
          n821 = call-poly "CoreLib.byte array 2 data.vi"("byteArray"=w1912, "error in (no error)"=w1913) -> ("i16"=w1903:i16, "error out"=w1910:errorcluster)  [unwired: 15 in, 1 out]
          n822 = Equal To 0?(x=w1903) -> (x = 0?=w1924:bool)
          n823 = Equal To 0?(x=w1894) -> (x = 0?=w1907:bool)
          n824 = Equal To 0?(x=w1900) -> (x = 0?=w1904:bool)
          n825 = Select(t=FALSE, s=w1924, f=TRUE) -> (s? t:f=w1902:bool)
          n826 = Select(t=FALSE, s=w1907, f=TRUE) -> (s? t:f=w1895:bool)
          n827 = Select(t=FALSE, s=w1904, f=TRUE) -> (s? t:f=w1901:bool)
          n828 = case shown="No Error" w1910 {
            tunnel: [w1951 w1956] -> w1931
            tunnel: w1936 -> [w1952 w1956]
            tunnel: w1935 -> [w1949 w1955]
            tunnel: [w1950 w1954] -> w1930
            tunnel: w1928 -> [_ w1953]
            tunnel: w1895 -> [w1948 _]
            tunnel: w1896 -> [w1947 _]
            tunnel: w1897 -> [w1946 _]
            tunnel: w1898 -> [w1945 _]
            tunnel: w1899 -> [w1944 _]
            tunnel: w1901 -> [w1943 _]
            tunnel: w1902 -> [w1942 _]
            frame No Error {
              # "Set?\nOutput\nMode\nAmplitude\nOffset\nInversion\nLoad"
              n829 = call "DG535.set outputs.vi"("i ref in"=w1952, "output"=w1947, "mode"=w1946, "amplitude"=w1945, "offset"=w1944, "error in (no error)"=w1949, "set"=w1948, "inversion"=w1943, "load"=w1942) -> ("i ref out"=w1951:refnum<vi>, "error out"=w1950:errorcluster)  [unwired: 9 in]
            }
            frame Error {
              n830 = call "CoreLib.set data type mismatch.vi"("error in (no error)"=w1955, "error source"=w1953) -> ("error out"=w1954:errorcluster)  [unwired: 17 in]
            }
          }
          n831 = call "BaseProcess.set event status.vi"("i ref in"=w1931, "EventStatus"=w1928, "error in (no error)"=w1930) -> ("i ref out"=w1927:refnum<vi>, "error out"=w1929:errorcluster)  [unwired: 14 in, 1 out]
          n832 = case shown="Error" w1929 {
            selector: w1929 -> [_ w1941]
            tunnel: [w1937 w1939] -> w1893
            frame No Error {
              n833 = call-poly "CoreLib.data 2 byte array.vi"("string"="" ("source")) -> ("byteArray out"=w1937:T1)  [unwired: 18 in]
            }
            frame Error {
              n834 = Unbundle By Name(w1941) -> ("source"=w1940:string)
              n835 = call-poly "CoreLib.data 2 byte array.vi"("string"=w1940) -> ("byteArray out"=w1939:T1)  [unwired: 18 in]
            }
          }
          n836 = Unbundle By Name(w1929) -> ("code"=w1934:i32)
          n837 = Bundle By Name(cluster=w1933, "Data"=w1893, "Error #"=w1934) -> (w1932:T2)
        }
        frame "GetActDelay" {
          n838 = call "DG535.GetActDelay.vi"("i ref in"=w1961, "error in (no error)"=w1962) -> ("i ref out"=w1960:refnum<vi>, "ActDelay"=w1959:dbl, "error out"=w1958:errorcluster)  [unwired: 15 in]
          n839 = call "BaseProcess.set event status.vi"("i ref in"=w1960, "EventStatus"=w1967, "error in (no error)"=w1958) -> ("i ref out"=w1963:refnum<vi>, "error out"=w1964:errorcluster)  [unwired: 14 in, 1 out]
          n840 = case shown="No Error" "error IO" {
            selector: "error IO" -> [_ w1975]
            tunnel: [w1971 w1973] -> w1968
            tunnel: w1959 -> [w1972 _]
            frame No Error {
              n841 = call-poly "CoreLib.data 2 byte array.vi"("f64"=w1972) -> ("byteArray out"=w1971:T1)  [unwired: 18 in]
            }
            frame Error {
              n842 = Unbundle By Name(w1975) -> ("source"=w1974:string)
              n843 = call-poly "CoreLib.data 2 byte array.vi"("string"=w1974) -> ("byteArray out"=w1973:T1)  [unwired: 18 in]
            }
          }
          n844 = Unbundle By Name(w1964) -> ("code"=w1970:i32)
          n845 = Bundle By Name(cluster=w1966, "Data"=w1968, "Error #"=w1970, "Data Descriptor"=T3 "D:1") -> (w1965:T2)
        }
        frame "GetADelay" {
          n846 = call "DG535.get A Delay.vi"("i ref in"=w1983, "error in (no error)"=w1982) -> ("i ref out"=w1980:refnum<vi>, "A"=w1979:dbl, "Ref Channel"=w1978:string, "error out"=w1981:errorcluster)  [unwired: 9 in, 1 out]
          n847 = call "BaseProcess.set event status.vi"("i ref in"=w1980, "EventStatus"=w1985, "error in (no error)"=w1981) -> ("i ref out"=w1984:refnum<vi>, "error out"=w1986:errorcluster)  [unwired: 14 in, 1 out]
          n848 = case shown="Error" w1986 {
            selector: w1986 -> [_ w1996]
            tunnel: [w1990 w1994] -> w1976
            tunnel: w1979 -> [w1992 _]
            tunnel: w1978 -> [w1993 _]
            frame No Error {
              n849 = call-poly "CoreLib.data 2 byte array.vi"("string"=w1993) -> ("byteArray out"=w1991:T1)  [unwired: 18 in]
              n850 = call-poly "CoreLib.data 2 byte array.vi"("byteArray"=w1991, "f64"=w1992) -> ("byteArray out"=w1990:T1)  [unwired: 17 in]
            }
            frame Error {
              n851 = Unbundle By Name(w1996) -> ("source"=w1995:string)
              n852 = call-poly "CoreLib.data 2 byte array.vi"("string"=w1995) -> ("byteArray out"=w1994:T1)  [unwired: 18 in]
            }
          }
          n853 = Unbundle By Name(w1986) -> ("code"=w1989:i32)
          n854 = Bundle By Name(cluster=w1988, "Data"=w1976, "Error #"=w1989, "Data Descriptor"=T3 "C:N;D:1") -> (w1987:T2)
        }
        frame "GetBDelay" {
          n855 = call "DG535.get B Delay.vi"("i ref in"=w2004, "error in (no error)"=w2003) -> ("i ref out"=w2001:refnum<vi>, "B"=w2000:dbl, "Ref Channel"=w1999:string, "error out"=w2002:errorcluster)  [unwired: 9 in, 1 out]
          n856 = call "BaseProcess.set event status.vi"("i ref in"=w2001, "EventStatus"=w2006, "error in (no error)"=w2002) -> ("i ref out"=w2005:refnum<vi>, "error out"=w2007:errorcluster)  [unwired: 14 in, 1 out]
          n857 = case shown="Error" w2007 {
            selector: w2007 -> [_ w2017]
            tunnel: [w2011 w2015] -> w1997
            tunnel: w2000 -> [w2013 _]
            tunnel: w1999 -> [w2014 _]
            frame No Error {
              n858 = call-poly "CoreLib.data 2 byte array.vi"("string"=w2014) -> ("byteArray out"=w2012:T1)  [unwired: 18 in]
              n859 = call-poly "CoreLib.data 2 byte array.vi"("byteArray"=w2012, "f64"=w2013) -> ("byteArray out"=w2011:T1)  [unwired: 17 in]
            }
            frame Error {
              n860 = Unbundle By Name(w2017) -> ("source"=w2016:string)
              n861 = call-poly "CoreLib.data 2 byte array.vi"("string"=w2016) -> ("byteArray out"=w2015:T1)  [unwired: 18 in]
            }
          }
          n862 = Unbundle By Name(w2007) -> ("code"=w2010:i32)
          n863 = Bundle By Name(cluster=w2009, "Data"=w1997, "Error #"=w2010, "Data Descriptor"=T3 "C:N;D:1") -> (w2008:T2)
        }
        frame "GetCDelay" {
          n864 = call "DG535.get C Delay.vi"("i ref in"=w2025, "error in (no error)"=w2024) -> ("i ref out"=w2022:refnum<vi>, "C"=w2021:dbl, "Ref Channel"=w2020:string, "error out"=w2023:errorcluster)  [unwired: 9 in, 1 out]
          n865 = call "BaseProcess.set event status.vi"("i ref in"=w2022, "EventStatus"=w2027, "error in (no error)"=w2023) -> ("i ref out"=w2026:refnum<vi>, "error out"=w2028:errorcluster)  [unwired: 14 in, 1 out]
          n866 = case shown="No Error" w2028 {
            selector: w2028 -> [_ w2038]
            tunnel: [w2032 w2036] -> w2019
            tunnel: w2021 -> [w2034 _]
            tunnel: w2020 -> [w2035 _]
            frame No Error {
              n867 = call-poly "CoreLib.data 2 byte array.vi"("string"=w2035) -> ("byteArray out"=w2033:T1)  [unwired: 18 in]
              n868 = call-poly "CoreLib.data 2 byte array.vi"("byteArray"=w2033, "f64"=w2034) -> ("byteArray out"=w2032:T1)  [unwired: 17 in]
            }
            frame Error {
              n869 = Unbundle By Name(w2038) -> ("source"=w2037:string)
              n870 = call-poly "CoreLib.data 2 byte array.vi"("string"=w2037) -> ("byteArray out"=w2036:T1)  [unwired: 18 in]
            }
          }
          n871 = Unbundle By Name(w2028) -> ("code"=w2031:i32)
          n872 = Bundle By Name(cluster=w2030, "Data"=w2019, "Error #"=w2031, "Data Descriptor"=T3 "C:N;D:1") -> (w2029:T2)
        }
        frame "GetDDelay" {
          n873 = call "DG535.get D Delay.vi"("i ref in"=w2045, "error in (no error)"=w2044) -> ("i ref out"=w2042:refnum<vi>, "D"=w2041:dbl, "Ref Channel"=w2040:string, "error out"=w2043:errorcluster)  [unwired: 9 in, 1 out]
          n874 = call "BaseProcess.set event status.vi"("i ref in"=w2042, "EventStatus"=w2047, "error in (no error)"=w2043) -> ("i ref out"=w2046:refnum<vi>, "error out"=w2048:errorcluster)  [unwired: 14 in, 1 out]
          n875 = case shown="No Error" w2048 {
            selector: w2048 -> [_ w2058]
            tunnel: [w2052 w2056] -> w2039
            tunnel: w2041 -> [w2054 _]
            tunnel: w2040 -> [w2055 _]
            frame No Error {
              n876 = call-poly "CoreLib.data 2 byte array.vi"("string"=w2055) -> ("byteArray out"=w2053:T1)  [unwired: 18 in]
              n877 = call-poly "CoreLib.data 2 byte array.vi"("byteArray"=w2053, "f64"=w2054) -> ("byteArray out"=w2052:T1)  [unwired: 17 in]
            }
            frame Error {
              n878 = Unbundle By Name(w2058) -> ("source"=w2057:string)
              n879 = call-poly "CoreLib.data 2 byte array.vi"("string"=w2057) -> ("byteArray out"=w2056:T1)  [unwired: 18 in]
            }
          }
          n880 = Unbundle By Name(w2048) -> ("code"=w2051:i32)
          n881 = Bundle By Name(cluster=w2050, "Data"=w2039, "Error #"=w2051) -> (w2049:T2)
        }
        frame "GetOutputsSettings" {
          n882 = Unbundle By Name(w2082) -> ("Data"=w2070:T1)
          n883 = call-poly "CoreLib.byte array 2 data.vi"("byteArray"=w2070) -> ("byteArray out"=w2069:T1, "i16"=w2062:i16, "error out"=w2068:errorcluster)  [unwired: 16 in]
          n884 = call-poly "CoreLib.byte array 2 data.vi"("byteArray"=w2069, "error in (no error)"=w2068) -> ("i32"=w2063:i32, "error out"=w2061:errorcluster)  [unwired: 15 in, 1 out]
          n885 = Equal To 0?(x=w2062) -> (x = 0?=w2065:bool)
          n886 = Select(t=FALSE, s=w2065, f=TRUE) -> (s? t:f=w2064:bool)
          n887 = case shown="No Error" w2061 {
            tunnel: [w2110 w2120] -> w2080
            tunnel: w2085 -> [w2111 w2120]
            tunnel: w2084 -> [w2108 w2119]
            tunnel: [w2109 w2118] -> w2079
            tunnel: w2063 -> [w2106 _]
            tunnel: w2077 -> [_ w2117]
            tunnel: w2064 -> [w2107 _]
            tunnel: [w2105 u8 0 ("mode")] -> w2075
            tunnel: [w2104 0.0 ("amplitude")] -> w2074
            tunnel: [w2103 0.0 ("offset")] -> w2073
            tunnel: [w2102 FALSE ("load")] -> w2072
            tunnel: [w2101 FALSE ("inversion")] -> w2071
            frame No Error {
              n888 = call "DG535.get outputs settings.vi"("i ref in"=w2111, "read"=w2107, "output"=w2106, "error in (no error)"=w2108) -> ("mode"=w2105:i32, "i ref out"=w2110:refnum<vi>, "amplitude"=w2104:dbl, "offset"=w2103:dbl, "load"=w2102:bool, "inversion"=w2101:bool, "error out"=w2109:errorcluster)  [unwired: 5 in]
            }
            frame Error {
              n889 = call "CoreLib.set data type mismatch.vi"("error in (no error)"=w2119, "error source"=w2117) -> ("error out"=w2118:errorcluster)  [unwired: 17 in]
            }
          }
          n890 = call "BaseProcess.set event status.vi"("i ref in"=w2080, "EventStatus"=w2077, "error in (no error)"=w2079) -> ("i ref out"=w2076:refnum<vi>, "error out"=w2078:errorcluster)  [unwired: 14 in, 1 out]
          n891 = case shown="No Error" w2078 {
            selector: w2078 -> [_ w2100]
            tunnel: [w2095 w2099] -> w2060
            tunnel: w2075 -> [w2087 _]
            tunnel: w2074 -> [w2088 _]
            tunnel: w2073 -> [w2090 _]
            tunnel: w2072 -> [w2097 _]
            tunnel: w2071 -> [w2096 _]
            frame No Error {
              n892 = call-poly "CoreLib.data 2 byte array.vi"("i32"=w2087) -> ("byteArray out"=w2086:T1)  [unwired: 18 in]
              n893 = Boolean To (0,1)(Boolean=w2097) -> (0, 1=w2093:i16)
              n894 = call-poly "CoreLib.data 2 byte array.vi"("byteArray"=w2086, "f64"=w2088) -> ("byteArray out"=w2089:T1)  [unwired: 17 in]
              n895 = Boolean To (0,1)(Boolean=w2096) -> (0, 1=w2094:i16)
              n896 = call-poly "CoreLib.data 2 byte array.vi"("byteArray"=w2089, "f64"=w2090) -> ("byteArray out"=w2091:T1)  [unwired: 17 in]
              n897 = call-poly "CoreLib.data 2 byte array.vi"("byteArray"=w2091, "i16"=w2093) -> ("byteArray out"=w2092:T1)  [unwired: 17 in]
              n898 = call-poly "CoreLib.data 2 byte array.vi"("byteArray"=w2092, "i16"=w2094) -> ("byteArray out"=w2095:T1)  [unwired: 17 in]
            }
            frame Error {
              n899 = Unbundle By Name(w2100) -> ("source"=w2098:string)
              n900 = call-poly "CoreLib.data 2 byte array.vi"("string"=w2098) -> ("byteArray out"=w2099:T1)  [unwired: 18 in]
            }
          }
          n901 = Unbundle By Name(w2078) -> ("code"=w2083:i32)
          n902 = Bundle By Name(cluster=w2082, "Data"=w2060, "Error #"=w2083, "Data Descriptor"=T3 "I:1;D:1;D:1;S:1;S:1") -> (w2081:T2)
        }
        frame "GetTriggerSlope" {
          n903 = call "DG535.get Trigger Slope.vi"("i ref in"=w2125, "error in (no error)"=w2126) -> ("i ref out"=w2124:refnum<vi>, "Tigger Slope"=w2122:bool, "error out"=w2123:errorcluster)  [unwired: 11 in]
          n904 = call "BaseProcess.set event status.vi"("i ref in"=w2124, "EventStatus"=w2128, "error in (no error)"=w2123) -> ("i ref out"=w2127:refnum<vi>, "error out"=w2129:errorcluster)  [unwired: 14 in, 1 out]
          n905 = case shown="No Error" w2129 {
            selector: w2129 -> [_ w2139]
            tunnel: [w2134 w2137] -> w2130
            tunnel: w2122 -> [w2136 _]
            frame No Error {
              n906 = Boolean To (0,1)(Boolean=w2136) -> (0, 1=w2135:i16)
              n907 = call-poly "CoreLib.data 2 byte array.vi"("i16"=w2135) -> ("byteArray out"=w2134:T1)  [unwired: 18 in]
            }
            frame Error {
              n908 = Unbundle By Name(w2139) -> ("source"=w2138:string)
              n909 = call-poly "CoreLib.data 2 byte array.vi"("string"=w2138) -> ("byteArray out"=w2137:T1)  [unwired: 18 in]
            }
          }
          n910 = Unbundle By Name(w2129) -> ("code"=w2133:i32)
          n911 = Bundle By Name(cluster=w2132, "Data"=w2130, "Error #"=w2133, "Data Descriptor"=T3 "S:1") -> (w2131:T2)
        }
        frame "GetInputImpedance" {
          n912 = call "DG535.get Input Impedance.vi"("i ref in"=w2144, "error in (no error)"=w2145) -> ("i ref out"=w2143:refnum<vi>, "Input Impedance"=w2141:bool, "error out"=w2142:errorcluster)  [unwired: 11 in]
          n913 = call "BaseProcess.set event status.vi"("i ref in"=w2143, "EventStatus"=w2147, "error in (no error)"=w2142) -> ("i ref out"=w2146:refnum<vi>, "error out"=w2148:errorcluster)  [unwired: 14 in, 1 out]
          n914 = case shown="No Error" w2148 {
            selector: w2148 -> [_ w2158]
            tunnel: [w2153 w2156] -> w2149
            tunnel: w2141 -> [w2155 _]
            frame No Error {
              n915 = Boolean To (0,1)(Boolean=w2155) -> (0, 1=w2154:i16)
              n916 = call-poly "CoreLib.data 2 byte array.vi"("i16"=w2154) -> ("byteArray out"=w2153:T1)  [unwired: 18 in]
            }
            frame Error {
              n917 = Unbundle By Name(w2158) -> ("source"=w2157:string)
              n918 = call-poly "CoreLib.data 2 byte array.vi"("string"=w2157) -> ("byteArray out"=w2156:T1)  [unwired: 18 in]
            }
          }
          n919 = Unbundle By Name(w2148) -> ("code"=w2152:i32)
          n920 = Bundle By Name(cluster=w2151, "Data"=w2149, "Error #"=w2152, "Data Descriptor"=T3 "S:1") -> (w2150:T2)
        }
        frame "GetExtTrigLevel" {
          n921 = call "DG535.get external trigger level.vi"("i ref in"=w2163, "error in (no error)"=w2164) -> ("i ref out"=w2162:refnum<vi>, "Ext Trig Level"=w2160:dbl, "error out"=w2161:errorcluster)  [unwired: 11 in]
          n922 = call "BaseProcess.set event status.vi"("i ref in"=w2162, "EventStatus"=w2166, "error in (no error)"=w2161) -> ("i ref out"=w2165:refnum<vi>, "error out"=w2167:errorcluster)  [unwired: 14 in, 1 out]
          n923 = case shown="No Error" w2167 {
            selector: w2167 -> [_ w2176]
            tunnel: [w2172 w2174] -> w2168
            tunnel: w2160 -> [w2173 _]
            frame No Error {
              n924 = call-poly "CoreLib.data 2 byte array.vi"("f64"=w2173) -> ("byteArray out"=w2172:T1)  [unwired: 18 in]
            }
            frame Error {
              n925 = Unbundle By Name(w2176) -> ("source"=w2175:string)
              n926 = call-poly "CoreLib.data 2 byte array.vi"("string"=w2175) -> ("byteArray out"=w2174:T1)  [unwired: 18 in]
            }
          }
          n927 = Unbundle By Name(w2167) -> ("code"=w2171:i32)
          n928 = Bundle By Name(cluster=w2170, "Data"=w2168, "Error #"=w2171, "Data Descriptor"=T3 "D:1") -> (w2169:T2)
        }
        frame "GetIntTrigRate" {
          n929 = call "DG535.get Internal trigger rate.vi"("i ref in"=w2181, "error in (no error)"=w2182) -> ("i ref out"=w2180:refnum<vi>, "Int Trigger Rate"=w2178:dbl, "error out"=w2179:errorcluster)  [unwired: 11 in]
          n930 = call "BaseProcess.set event status.vi"("i ref in"=w2180, "EventStatus"=w2184, "error in (no error)"=w2179) -> ("i ref out"=w2183:refnum<vi>, "error out"=w2185:errorcluster)  [unwired: 14 in, 1 out]
          n931 = case shown="No Error" w2185 {
            selector: w2185 -> [_ w2194]
            tunnel: [w2190 w2192] -> w2186
            tunnel: w2178 -> [w2191 _]
            frame No Error {
              n932 = call-poly "CoreLib.data 2 byte array.vi"("f64"=w2191) -> ("byteArray out"=w2190:T1)  [unwired: 18 in]
            }
            frame Error {
              n933 = Unbundle By Name(w2194) -> ("source"=w2193:string)
              n934 = call-poly "CoreLib.data 2 byte array.vi"("string"=w2193) -> ("byteArray out"=w2192:T1)  [unwired: 18 in]
            }
          }
          n935 = Unbundle By Name(w2185) -> ("code"=w2189:i32)
          n936 = Bundle By Name(cluster=w2188, "Data"=w2186, "Error #"=w2189, "Data Descriptor"=T3 "D:1") -> (w2187:T2)
        }
        frame "GetBurstTrigRate" {
          n937 = call "DG535.get burst trigger rate.vi"("i ref in"=w2199, "error in (no error)"=w2200) -> ("i ref out"=w2198:refnum<vi>, "Burst Trig Rate"=w2196:dbl, "error out"=w2197:errorcluster)  [unwired: 11 in]
          n938 = call "BaseProcess.set event status.vi"("i ref in"=w2198, "EventStatus"=w2202, "error in (no error)"=w2197) -> ("i ref out"=w2201:refnum<vi>, "error out"=w2203:errorcluster)  [unwired: 14 in, 1 out]
          n939 = case shown="No Error" w2203 {
            selector: w2203 -> [_ w2212]
            tunnel: [w2208 w2210] -> w2204
            tunnel: w2196 -> [w2209 _]
            frame No Error {
              n940 = call-poly "CoreLib.data 2 byte array.vi"("f64"=w2209) -> ("byteArray out"=w2208:T1)  [unwired: 18 in]
            }
            frame Error {
              n941 = Unbundle By Name(w2212) -> ("source"=w2211:string)
              n942 = call-poly "CoreLib.data 2 byte array.vi"("string"=w2211) -> ("byteArray out"=w2210:T1)  [unwired: 18 in]
            }
          }
          n943 = Unbundle By Name(w2203) -> ("code"=w2207:i32)
          n944 = Bundle By Name(cluster=w2206, "Data"=w2204, "Error #"=w2207, "Data Descriptor"=T3 "D:1") -> (w2205:T2)
        }
        frame "GetBurstCount" {
          n945 = call "DG535.get burst count.vi"("i ref in"=w2218, "error in (no error)"=w2219) -> ("i ref out"=w2217:refnum<vi>, "Burst Count"=w2215:i32, "error out"=w2216:errorcluster)  [unwired: 11 in]
          n946 = call "BaseProcess.set event status.vi"("i ref in"=w2217, "EventStatus"=w2221, "error in (no error)"=w2216) -> ("i ref out"=w2220:refnum<vi>, "error out"=w2222:errorcluster)  [unwired: 14 in, 1 out]
          n947 = case shown="No Error" w2222 {
            selector: w2222 -> [_ w2230]
            tunnel: [w2226 w2228] -> w2214
            tunnel: w2215 -> [w2227 _]
            frame No Error {
              n948 = call-poly "CoreLib.data 2 byte array.vi"("i32"=w2227) -> ("byteArray out"=w2226:T1)  [unwired: 18 in]
            }
            frame Error {
              n949 = Unbundle By Name(w2230) -> ("source"=w2229:string)
              n950 = call-poly "CoreLib.data 2 byte array.vi"("string"=w2229) -> ("byteArray out"=w2228:T1)  [unwired: 18 in]
            }
          }
          n951 = Unbundle By Name(w2222) -> ("code"=w2225:i32)
          n952 = Bundle By Name(cluster=w2224, "Data"=w2214, "Error #"=w2225, "Data Descriptor"=T3 "I:1") -> (w2223:T2)
        }
        frame "GetBurstPeriod" {
          n953 = call "DG535.get burst period.vi"("i ref in"=w2236, "error in (no error)"=w2237) -> ("i ref out"=w2235:refnum<vi>, "Burst Period"=w2233:i32, "error out"=w2234:errorcluster)  [unwired: 11 in]
          n954 = call "BaseProcess.set event status.vi"("i ref in"=w2235, "EventStatus"=w2239, "error in (no error)"=w2234) -> ("i ref out"=w2238:refnum<vi>, "error out"=w2240:errorcluster)  [unwired: 14 in, 1 out]
          n955 = case shown="No Error" w2240 {
            selector: w2240 -> [_ w2248]
            tunnel: [w2244 w2246] -> w2232
            tunnel: w2233 -> [w2245 _]
            frame No Error {
              n956 = call-poly "CoreLib.data 2 byte array.vi"("i32"=w2245) -> ("byteArray out"=w2244:T1)  [unwired: 18 in]
            }
            frame Error {
              n957 = Unbundle By Name(w2248) -> ("source"=w2247:string)
              n958 = call-poly "CoreLib.data 2 byte array.vi"("string"=w2247) -> ("byteArray out"=w2246:T1)  [unwired: 18 in]
            }
          }
          n959 = Unbundle By Name(w2240) -> ("code"=w2243:i32)
          n960 = Bundle By Name(cluster=w2242, "Data"=w2232, "Error #"=w2243, "Data Descriptor"=T3 "I:1") -> (w2241:T2)
        }
        frame "GetTriggerMode" {
          n961 = call "DG535.get trigger mode.vi"("i ref in"=w2254, "error in (no error)"=w2255) -> ("i ref out"=w2253:refnum<vi>, "Trigger Mode"=w2251:u32, "error out"=w2252:errorcluster)  [unwired: 11 in]
          n962 = call "BaseProcess.set event status.vi"("i ref in"=w2253, "EventStatus"=w2257, "error in (no error)"=w2252) -> ("i ref out"=w2256:refnum<vi>, "error out"=w2258:errorcluster)  [unwired: 14 in, 1 out]
          n963 = case shown="No Error" w2258 {
            selector: w2258 -> [_ w2266]
            tunnel: [w2262 w2264] -> w2250
            tunnel: w2251 -> [w2263 _]
            frame No Error {
              n964 = call-poly "CoreLib.data 2 byte array.vi"("i32"=w2263) -> ("byteArray out"=w2262:T1)  [unwired: 18 in]
            }
            frame Error {
              n965 = Unbundle By Name(w2266) -> ("source"=w2265:string)
              n966 = call-poly "CoreLib.data 2 byte array.vi"("string"=w2265) -> ("byteArray out"=w2264:T1)  [unwired: 18 in]
            }
          }
          n967 = Unbundle By Name(w2258) -> ("code"=w2261:i32)
          n968 = Bundle By Name(cluster=w2260, "Data"=w2250, "Error #"=w2261, "Data Descriptor"=T3 "I:1") -> (w2259:T2)
        }
      }
    }
    frame Error {
    }
  }
  "answer cluster" <- w7
  "i ref out" <- w4
  "error out" <- w3
